vi "运维调试_五参数.vi"(11 "编号":string) -> ()   [LabVIEW 2016, in "斯坦道多参数.lvlib"]
uses:
  <vilib>/Utility/miscctls.llb/LVPointTypeDef.ctl
  <vilib>/Plasmionique/MB Master/MB_Master/MB_Master.lvclass
  <vilib>/Utility/config.llb/NI_LVConfig.lvlib
panel:
  in  "水样测量时间":dbl caption="水样测量时间:"
  in  "自动断线重连":bool=TRUE
  in  "打开modbus":bool
  out "选项卡控件":enum32{"选项卡 1", "选项卡 2"}(tab)
  in  "VISA资源名称":refnum<visa-resource-name> caption="串口"
  in  "IP":string="localhost" caption="IP:"
  in  "Port":u16=502 caption="Port:"
  in  "连接方式":u16(ring) items=["Modbus RTU", "Modbus TCP"]
  in  "藻密度校准":bool
  in  "权限2":bool
  out "权限1":bool
  out "密码":dbl
  in  "密码锁":bool
  in  "藻密度探头选择":u16(ring) items=["YL型", "MQ型", "NAQ型"]
  in  "叶绿素a探头选择":u16(ring) items=["YL型", "MQ型", "NAQ型"]
  in  "浊度探头选择":u16(ring) items=["YL型", "MQ型", "NAQ型"]
  in  "电导率探头选择":u16(ring) items=["YL型", "MQ型", "NAQ型"]
  in  "DO探头选择":u16(ring) items=["YL型", "MQ型", "NAQ型"]
  in  "pH探头选择":u16(ring) items=["YL型", "MQ型", "NAQ型"]
  in  "设置页返回":bool
  in  "藻密度":bool
  in  "叶绿素a启用":bool
  in  "Temp":bool
  in  "Cond":bool
  in  "Turb":bool
  in  "DO":bool
  in  "pH":bool
  in  "周期设置":bool
  out "当前串口":string
  out "运行状态":u16(ring) items=["空闲", "水样测试", "标样核查"]
  in  "叶绿素a校准":bool
  in  "停止":bool
  in  "标样核查":bool
  in  "水样测试":bool
  in  "设置":bool
  in  "水温校准":bool
  in  "浊度校准":bool
  in  "溶解氧校准":bool
  in  "电导率校准":bool
  in  "pH校准":bool
  in  "探头校正返回":bool
  in  "探头校正":bool
  out "检测值":T1(array[cluster])
  # "请设置仪器连接方式"
  # "请选择要启用的参数"
  # "min"
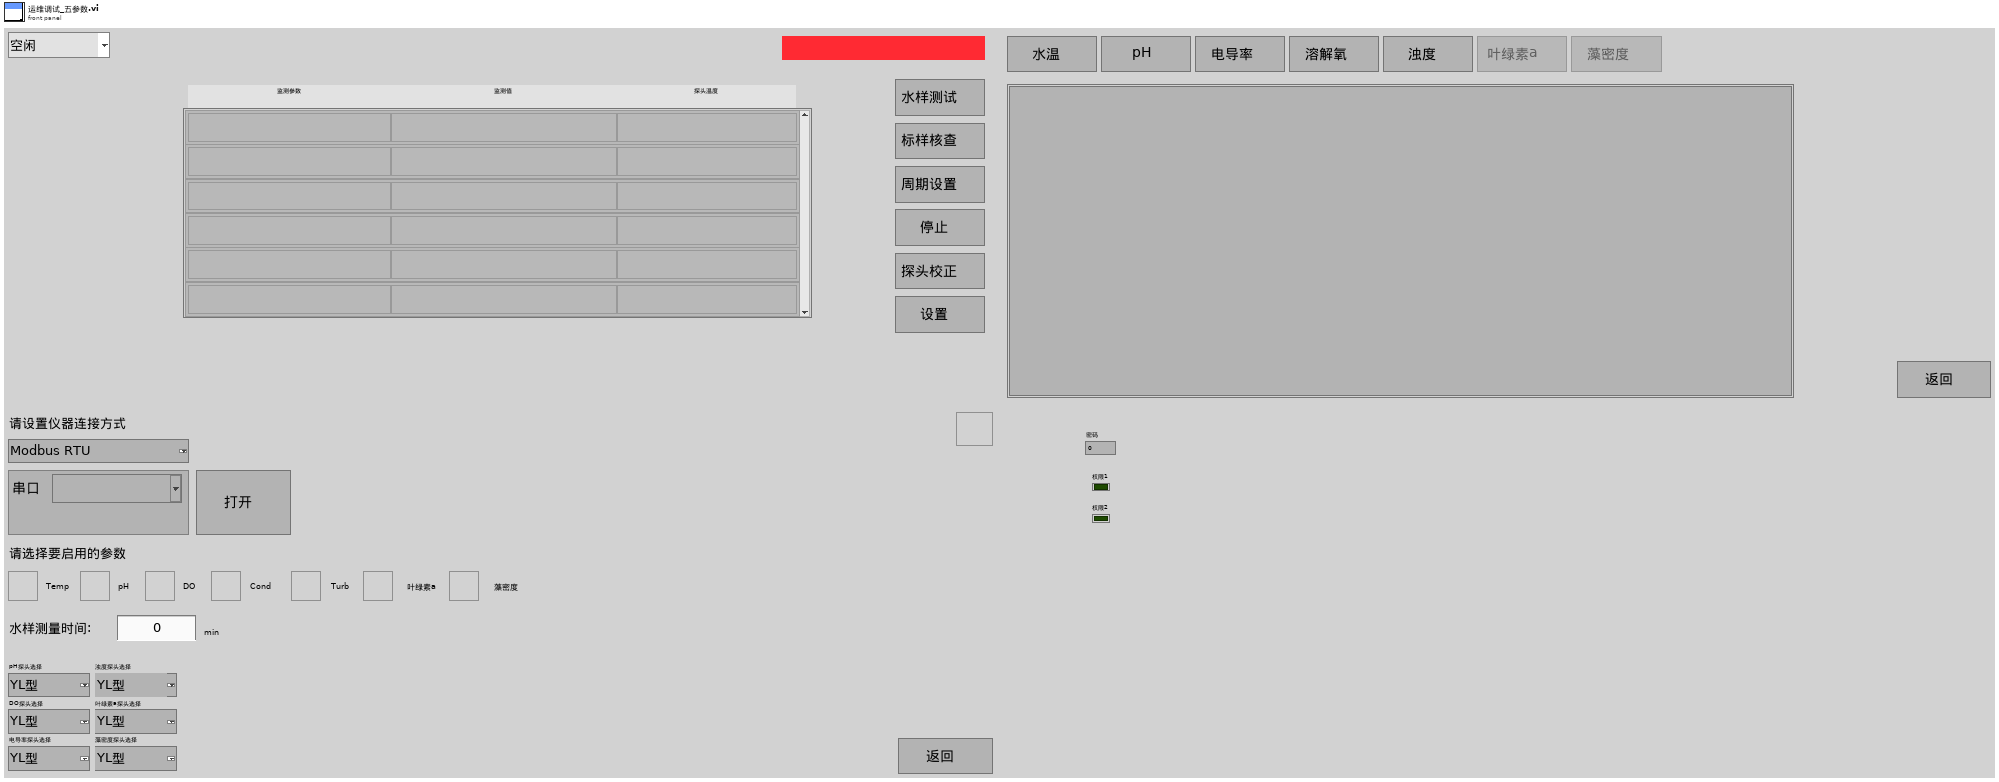
[diagram p1: front panel]
types:
  T1 = cluster{"监测参数1":string, "浓度1":string, "探头温度1":string}[]
  T2 = typedef "LVPointTypeDef.ctl" = cluster{"Horizontal":i16, "Vertical":i16}
  T3 = cluster{"温度测量值":sgl, "DO%":sgl, "DOmg/L":sgl, "温度偏移修正值":sgl}
  T4 = enum8{"Enabled", "Disabled", "Disabled and Grayed Out"}
  T5 = cluster{"pH探头选择":u16, "DO探头选择":u16, "电导率探头选择":u16, "浊度探头选择":u16, "叶绿素a探头选择":u16, "蓝绿藻探头选择":u16}
  T6 = cluster{"周期设置类型":enum16{"定点启动", "间隔启动"}, "定时功能启用":bool, "定时间隔":u32, "24H周期设置":bool[]}
  T7 = enum32{"Bad", "Idle", "Run top level", "Running"}
  T8 = typedef "LVDateTimeRec.ctl" = cluster{"秒数的小数部分":dbl, "秒":i32, "分":i32, "时":i32, "日":i32, "月":i32, "年":i32, "天数（周）":i32, "天数（年）":i32, "DST":i32}
  T9 = typedef "Semaphore RefNum" = refnum<k1>
  T10 = cluster{"电极状态标志":u16, "电极型号标志":u16, "溶解氧测量值":sgl, "温度测量值":sgl, "溶解氧饱和度值":sgl, "盐度补偿值":sgl, "大气压补偿值":sgl, "溶解氧偏移修正值":sgl, "温度偏移修正值":sgl, "手动温度补偿值":sgl, "溶解氧电极零点":sgl, "溶解氧电极斜率":sgl, "第1点标准值记录":sgl, "第1点信号值记录":sgl, "第1点温度值记录":sgl, "第2点标准值记录":sgl, "第2点信号值记录":sgl, "第2点温度值记录":sgl, "命令滤波设定":u16, "温度模式":enum16{"ATC", "MTC"}, "生产批次":u16, "电极序号":u16, "串口地址":u16, "串口波特率":enum16{"9600", "19200", "115200"}, "串口校验位":enum16{"NONE", "ODD", "EVEN"}, "串口停止位":enum16{"1bit", "2bit"}, "第一点标准值":sgl, "第二点标准值":sgl}
  T11 = cluster{"报警码":u16, "溶解氧数值（mg/L）":sgl, "溶解氧数据（%）":sgl, "温度数据":sgl, "溶解氧原始信号 nA":sgl, "大气压力":sgl, "盐度":sgl, "0X0009_NC":string, "产品名称":string, "序列号":string, "硬件版本":string, "软件版本":string, "通讯地址":u16, "波特率":u16, "设备类型":u16, "0X0026_NC":string, "第一点原始数据":sgl, "0X0033 NC":sgl, "第二点原始数据":sgl, "0X0037 NC":sgl, "探头校准命令":u16, "温度校准参数":sgl, "温度校准命令":u16}
  T12 = cluster{"电极状态标志":u16, "电极型号标志":u16, "酸碱度测量值":sgl, "温度测量值":sgl, "酸碱度信号值":sgl, "温度信号值":sgl, "酸碱度偏移修正值":sgl, "温度偏移修正值":sgl, "手动温度补偿值":sgl, "酸碱度电极零点":sgl, "酸碱度电极斜率":sgl, "第1点标准值记录":sgl, "第1点信号值记录":sgl, "第1点温度值记录":sgl, "第2点标准值记录":sgl, "第2点信号值记录":sgl, "第2点温度值记录":sgl, "命令滤波设定":u16, "温度模式":enum16{"ATC", "MTC"}, "生产批次":u16, "电极序号":u16, "串口地址":u16, "串口波特率":enum16{"9600", "19200", "115200"}, "串口校验位":enum16{"NONE", "ODD", "EVEN"}, "串口停止位":enum16{"1bit", "2bit"}, "第一点标准值":sgl, "第二点标准值":sgl}
  T13 = cluster{"报警码":u16, "pH数值":sgl, "0X0003_NC":sgl, "温度数据":sgl, "pH原始信号 mv":sgl, "0X0009_NC":string, "产品名称":string, "序列号":string, "硬件版本":string, "软件版本":string, "通讯地址":u16, "波特率":u16, "设备类型":u16, "0X0026_NC":string, "第一点原始数据":sgl, "第一点校准数据":sgl, "第二点原始数据":sgl, "第二点校准数据":sgl, "探头校准命令":u16, "温度校准参数":sgl, "温度校准命令":u16}
  T14 = cluster{"电极状态标志":u16, "电极型号标志":u16, "浊度测量值":sgl, "温度测量值":sgl, "浊度信号值":sgl, "浊度偏移修正值":sgl, "温度偏移修正值":sgl, "手动温度补偿值":sgl, "浊度电极零点":sgl, "浊度电极斜率":sgl, "第1点标准值记录":sgl, "第1点信号值记录":sgl, "第1点温度值记录":sgl, "第2点标准值记录":sgl, "第2点信号值记录":sgl, "第2点温度值记录":sgl, "命令滤波设定":u16, "温度模式":enum16{"ATC", "MTC"}, "生产批次":u16, "电极序号":u16, "串口地址":u16, "串口波特率":enum16{"9600", "19200", "115200"}, "串口校验位":enum16{"NONE", "ODD", "EVEN"}, "串口停止位":enum16{"1bit", "2bit"}, "第一点标准值":sgl, "第二点标准值":sgl, "第三点标准值":sgl}
  T15 = cluster{"报警码":u16, "浊度数值 NTU":sgl, "温度数据":sgl, "原始光强数值":u16, "量程":u16, "平均次数":u16, "清扫模式":u16, "清扫次数":u16, "清扫间隔分钟":u16, "0X000B_NC":string, "产品名称":string, "序列号":string, "硬件版本":string, "软件版本":string, "通讯地址":u16, "波特率":u16, "设备类型":u16, "0X0026_NC":string, "校准量程":u16, "第一点原始光强":u16, "第一点校准数据":sgl, "第二点原始光强":u16, "第二点校准数据":sgl, "第三点原始光强":u16, "第三点校准数据":sgl, "探头校准命令":u16, "温度校准参数":sgl, "温度校准命令":u16}
  T16 = cluster{"报警码":u16, "蓝绿藻":sgl, "温度数据":sgl, "原始光强数值":u16, "0X0006_NC":u16, "平均次数":u16, "清扫模式":u16, "清扫次数":u16, "清扫间隔分钟":u16, "0X000B_NC":string, "产品名称":string, "序列号":string, "硬件版本":string, "软件版本":string, "通讯地址":u16, "波特率":u16, "设备类型":u16, "0X0026_NC":string, "0X0030_NC":u16, "第一点原始光强":u16, "第一点校准数据":sgl, "第二点原始光强":u16, "第二点校准数据":sgl, "第三点原始光强":u16, "第三点校准数据":sgl, "探头校准命令":u16, "温度校准参数":sgl, "温度校准命令":u16}
  T17 = cluster{"报警码":u16, "叶绿素a":sgl, "温度数据":sgl, "原始光强数值":u16, "0X0006_NC":u16, "平均次数":u16, "清扫模式":u16, "清扫次数":u16, "清扫间隔分钟":u16, "0X000B_NC":string, "产品名称":string, "序列号":string, "硬件版本":string, "软件版本":string, "通讯地址":u16, "波特率":u16, "设备类型":u16, "0X0026_NC":string, "0X0030_NC":u16, "第一点原始光强":u16, "第一点校准数据":sgl, "第二点原始光强":u16, "第二点校准数据":sgl, "第三点原始光强":u16, "第三点校准数据":sgl, "探头校准命令":u16, "温度校准参数":sgl, "温度校准命令":u16}
  T18 = cluster{"电极状态标志":u16, "电极型号标志":u16, "电导率测量值":sgl, "温度测量值":sgl, "电导率信号值":sgl, "温度信号值":sgl, "温度补偿系数":sgl, "电导率偏移修正值":sgl, "温度偏移修正值":sgl, "手动温度补偿值":sgl, "电导率电极零点":sgl, "电导率电极斜率":sgl, "命令滤波设定":u16, "温度模式":enum16{"ATC", "MTC"}, "生产批次":u16, "电极序号":u16, "串口地址":u16, "串口波特率":enum16{"9600", "19200", "115200"}, "串口校验位":enum16{"NONE", "ODD", "EVEN"}, "串口停止位":enum16{"1bit", "2bit"}, "第一点标准值":sgl, "第二点标准值":sgl}
  T19 = cluster{"报警码":u16, "电导率数据（uS/cm）":sgl, "0x0003 NC":sgl, "温度数据":sgl, "电导率原始信号电阻":sgl, "当前量程":u16, "温度补偿系数":sgl, "0X0009_NC":string, "产品名称":string, "序列号":string, "硬件版本":string, "软件版本":string, "通讯地址":u16, "波特率":u16, "设备类型":u16, "0X0026_NC":string, "第一点原始数据":sgl, "第一点校准数据":sgl, "0X0035_NC":sgl, "0X0037_NC":sgl, "探头校准命令":u16, "温度校准参数":sgl, "温度校准命令":u16}
  T20 = typedef "NI_LVConfig.lvlib/Config Data RefNum.ctl" = refnum<k1>
  T21 = cluster{"pH校准VI引用句柄":refnum<vi>, "DO校准VI引用句柄":refnum<vi>, "COND校准VI引用句柄":refnum<vi>, "TURB校准VI引用句柄":refnum<vi>, "CHLA校准VI引用句柄":refnum<vi>, "BGA校准VI引用句柄":refnum<vi>}
  T22 = cluster{"数据保存间隔":dbl, "水温标样值":dbl, "pH标样值":dbl, "溶解氧标样值":dbl, "电导率标样值":dbl, "浊度标样值":dbl}
  T23 = cluster{"baud rate (bps)":u32, "stop bits":u16, "parity":u16, "flow control":u16, "timeout":u32, "retries":i32}
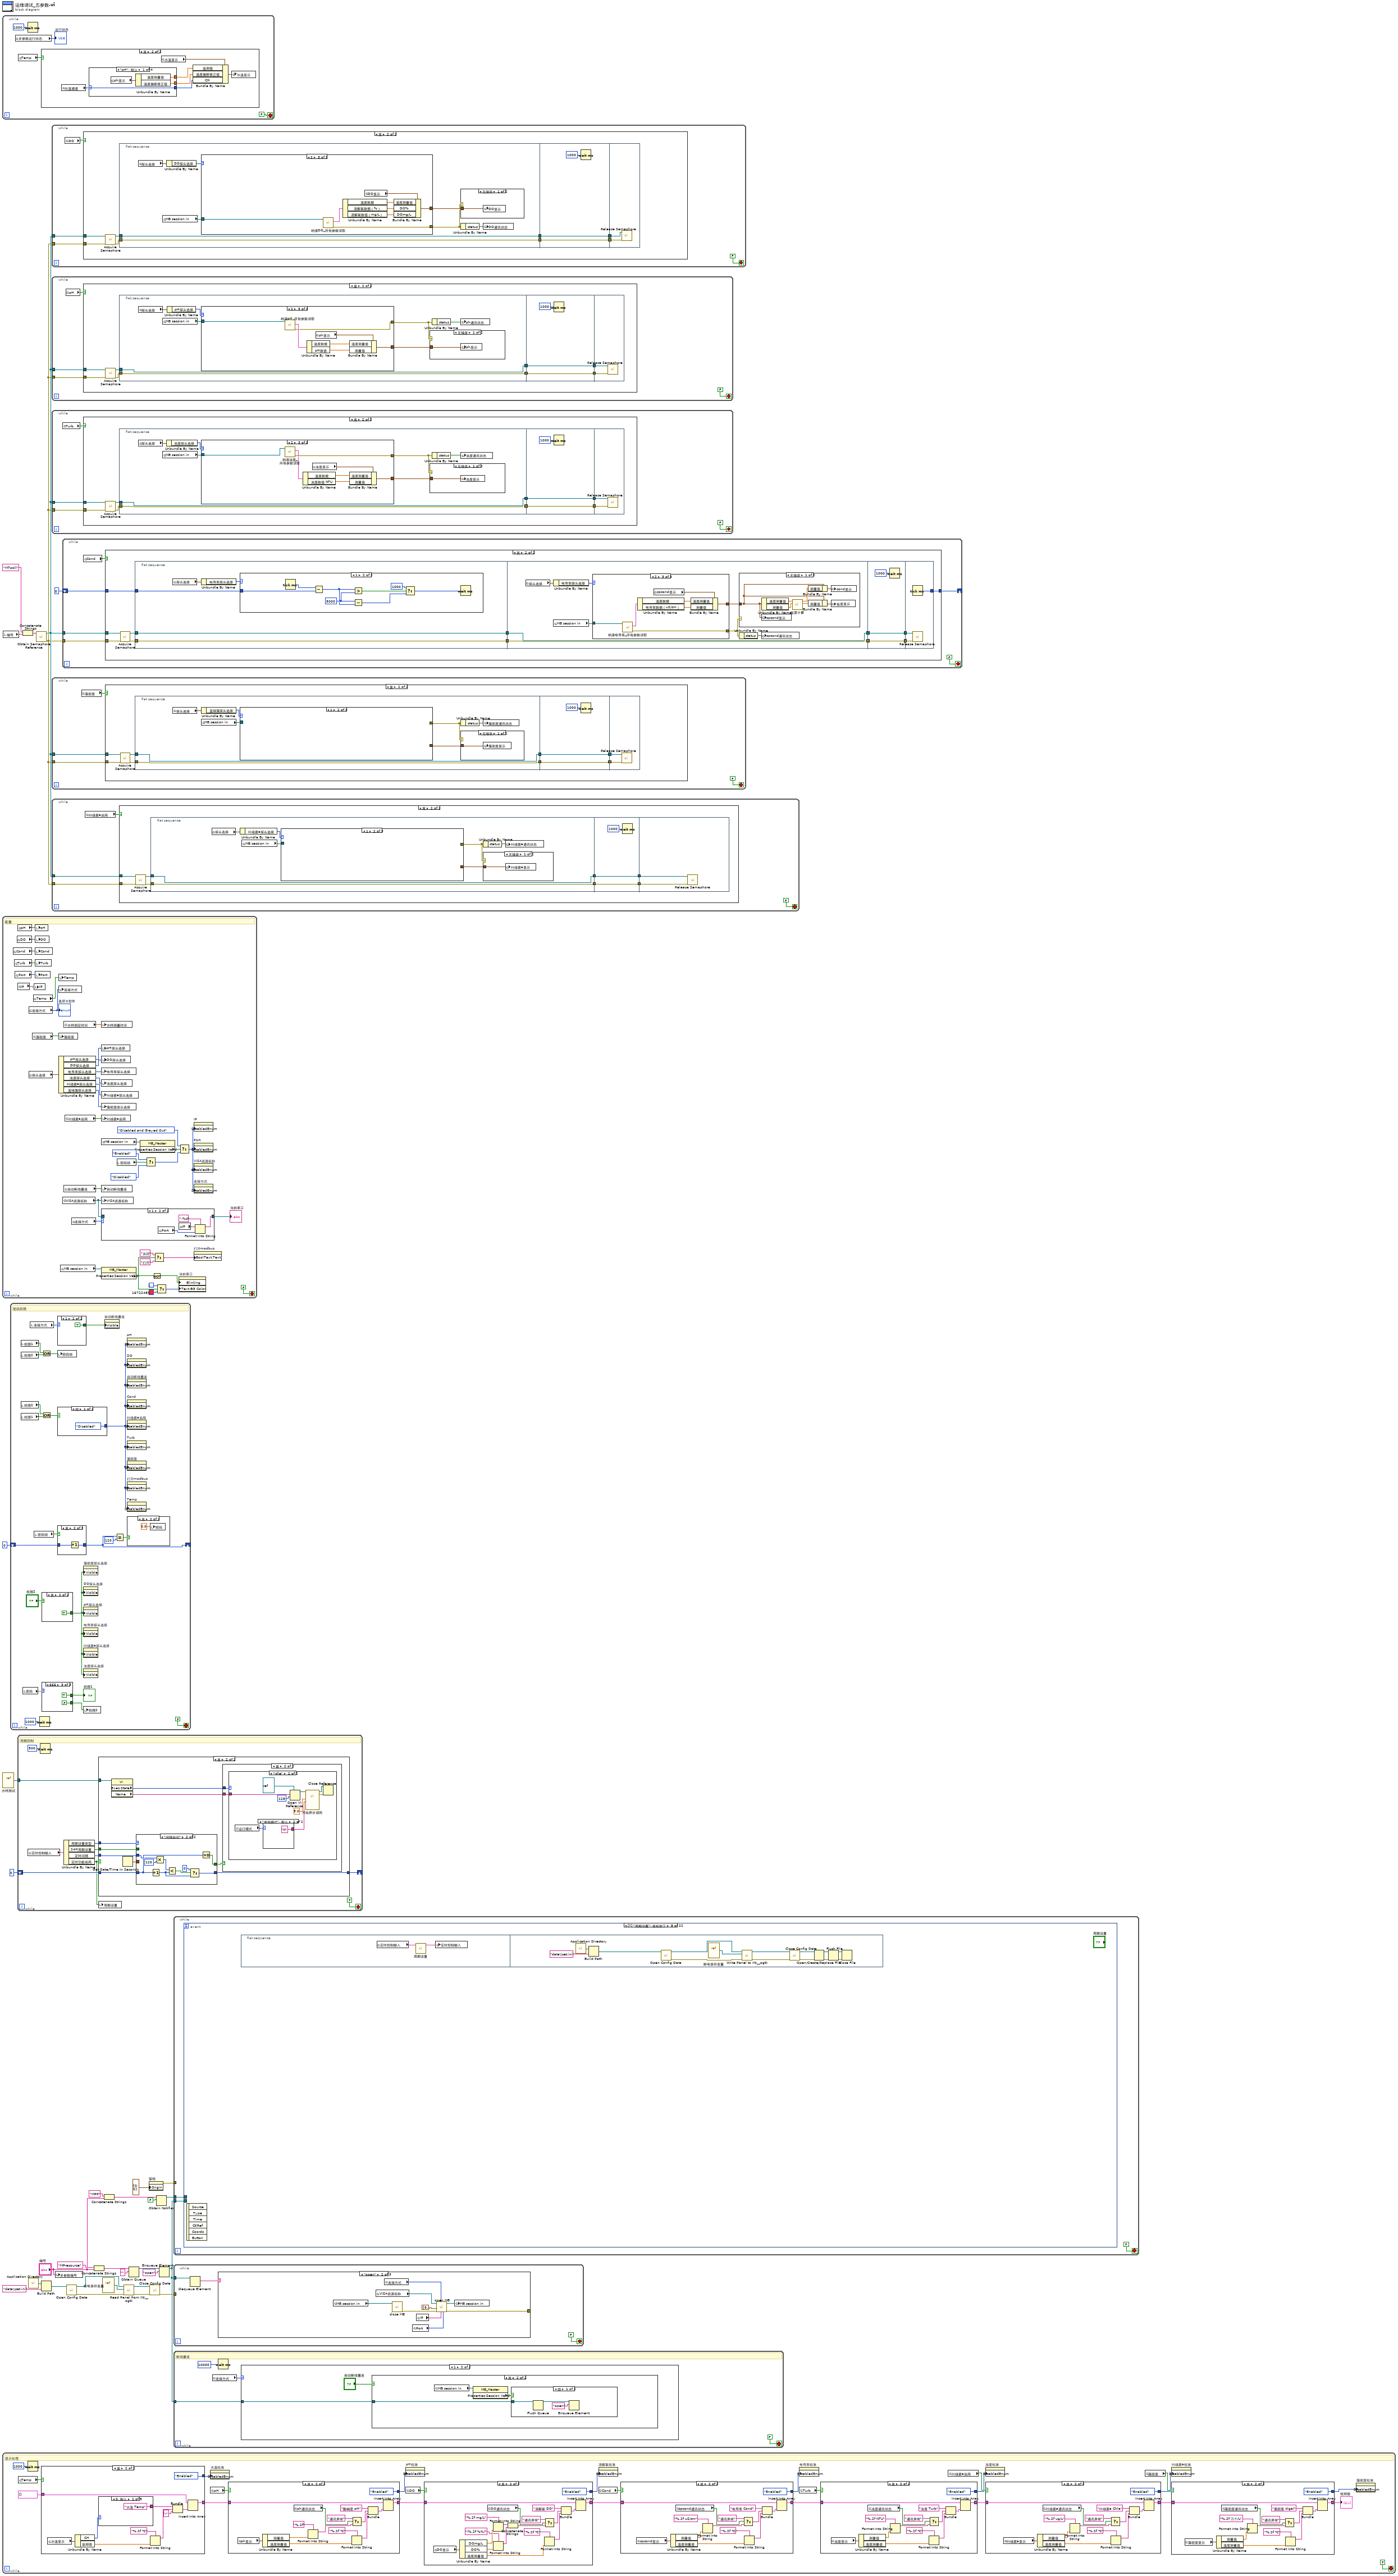
[diagram p0: block diagram]
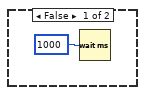
[diagram p5: hidden frame]
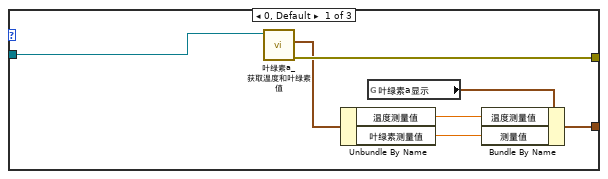
[diagram p6: hidden frame]
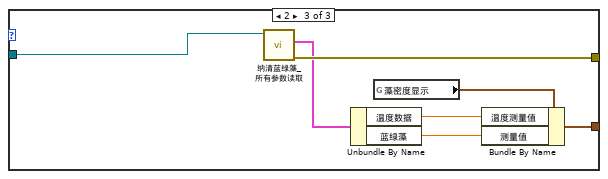
[diagram p7: hidden frame]
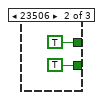
[diagram p13: hidden frame]
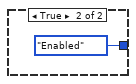
[diagram p14: hidden frame]
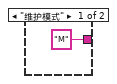
[diagram p19: hidden frame]
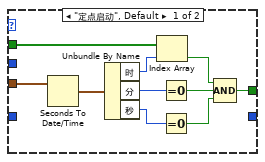
[diagram p20: hidden frame]
diagram:
  n1 = while {
    stop <- FALSE stop-if-true
    n2 = global read "多参数全局变量.vi" "多参数运行状态"() -> (→"运行状态":u16)
    n3 = global read "断电保存变量.vi" "Temp"() -> (w33:bool)
    n4 = Wait (ms)(milliseconds to wait=u32 1000 ("等待时间（毫秒）")) -> ()  [unwired: 1 out]
    n5 = case shown="真" w33 {
      frame False {
      }
      frame True {
        n6 = global read "断电保存变量.vi" "水温通道"() -> (w41:enum16{"pH", "Cond", "DO", "Turb"})
        n7 = case shown="\"pH\", 默认" w41 {
          selector: w41 -> [w45 w49 w53 w57]
          tunnel: [w45 w49 w53 w57] -> w40
          tunnel: [w43 w46 w50 w54] -> w39
          tunnel: [w44 w47 w51 w55] -> w38
          frame "pH", Default {
            n8 = global read "多参数全局变量.vi" "ph显示"() -> (w42:cluster{"温度测量值":sgl, "测量值":sgl, "温度偏移修正值":sgl})
            n9 = Unbundle By Name(w42) -> ("温度测量值"=w44:sgl, "温度偏移修正值"=w43:sgl)
          }
          frame "Cond" {
            n10 = global read "多参数全局变量.vi" "spcond显示"() -> (w48:cluster{"温度测量值":sgl, "测量值":sgl, "温度偏移修正值":sgl})
            n11 = Unbundle By Name(w48) -> ("温度测量值"=w47:sgl, "温度偏移修正值"=w46:sgl)
          }
          frame "DO" {
            n12 = global read "多参数全局变量.vi" "DO显示"() -> (w52:T3)
            n13 = Unbundle By Name(w52) -> ("温度测量值"=w51:sgl, "温度偏移修正值"=w50:sgl)
          }
          frame "Turb" {
            n14 = global read "多参数全局变量.vi" "浊度显示"() -> (w56:cluster{"温度测量值":sgl, "测量值":sgl, "温度偏移修正值":sgl})
            n15 = Unbundle By Name(w56) -> ("温度测量值"=w55:sgl, "温度偏移修正值"=w54:sgl)
          }
        }
        n16 = global read "多参数全局变量.vi" "水温显示"() -> (w36:cluster{"CH":u16, "监测值":dbl, "温度偏移修正值":sgl})
        n17 = Bundle By Name(cluster=w36, "监测值"=w38, "温度偏移修正值"=w39, "CH"=w40) -> (w37:cluster{"CH":u16, "监测值":dbl, "温度偏移修正值":sgl})
        n18 = global write "多参数全局变量.vi" "水温显示"(w37) -> ()
      }
    }
  }
  n19 = while {
    stop <- FALSE stop-if-true
    # "配置"
    n20 = global read "断电保存变量.vi" "Cond"() -> (w93:bool)
    n21 = global read "断电保存变量.vi" "Turb"() -> (w92:bool)
    n22 = global read "断电保存变量.vi" "Port"() -> (w71:u16)
    n23 = global read "断电保存变量.vi" "DO"() -> (w94:bool)
    n24 = global read "断电保存变量.vi" "pH"() -> (w95:bool)
    n25 = global read "断电保存变量.vi" "IP"() -> (w72:string)
    n26 = global read "断电保存变量.vi" "连接方式"() -> (w64:u16)
    "选项卡控件" <- w64
    n27 = global read "断电保存变量.vi" "探头选择"() -> (w82:T5)
    n28 = global read "断电保存变量.vi" "藻密度"() -> (w90:bool)
    n29 = global read "断电保存变量.vi" "Temp"() -> (w96:bool)
    n30 = local write "IP"(w72) -> ()
    n31 = local write "pH"(w95) -> ()
    n32 = local write "DO"(w94) -> ()
    n33 = local write "Cond"(w93) -> ()
    n34 = local write "Turb"(w92) -> ()
    n35 = local write "Port"(w71) -> ()
    n36 = local write "Temp"(w96) -> ()
    n37 = local write "连接方式"(w64) -> ()
    n38 = local write "藻密度"(w90) -> ()
    n39 = Unbundle By Name(w82) -> ("pH探头选择"=w65:u16, "DO探头选择"=w81:u16, "电导率探头选择"=w80:u16, "浊度探头选择"=w79:u16, "叶绿素a探头选择"=w78:u16, "蓝绿藻探头选择"=w77:u16)
    n40 = global read "多参数全局变量.vi" "MB session in"() -> (w86:refnum<class "MB_Master.lvclass">)
    n41 = global read "断电保存变量.vi" "VISA资源名称"() -> (w68:refnum<visa-resource-name>)
    n42 = global read "断电保存变量.vi" "水样测定时间"() -> (w58:dbl)
    n43 = global read "断电保存变量.vi" "自动断线重连"() -> (w59:bool)
    n44 = global read "断电保存变量.vi" "叶绿素a启用"() -> (w91:bool)
    n45 = global read "断电保存变量.vi" "连接方式"() -> (w69:u16)
    n46 = local write "水样测量时间"(w58) -> ()
    n47 = local write "pH探头选择"(w65) -> ()
    n48 = local write "DO探头选择"(w81) -> ()
    n49 = local write "电导率探头选择"(w80) -> ()
    n50 = local write "浊度探头选择"(w79) -> ()
    n51 = local write "叶绿素a探头选择"(w78) -> ()
    n52 = local write "藻密度探头选择"(w77) -> ()
    n53 = local write "叶绿素a启用"(w91) -> ()
    n54 = global read "多参数全局变量.vi" "MB session in"() -> (w89:refnum<class "MB_Master.lvclass">)
    n55 = local write "自动断线重连"(w59) -> ()
    n56 = local write "VISA资源名称"(w68) -> ()
    n57 = case shown="1" w69 {
      tunnel: w68 -> [w98 _]
      tunnel: [w98 w99] -> w67
      frame 0, Default {
      }
      frame 1 {
        n58 = global read "断电保存变量.vi" "Port"() -> (w100:u16)
        n59 = global read "断电保存变量.vi" "IP"() -> (w102:string)
        n60 = Format Into String(format string=":%d" ("格式字符串"), initial string=w102, w100) -> (resulting string=w99:string)  [unwired: 1 in, 1 out]
      }
    }
    "当前串口" <- w67
    n61 = property class="MB_Master"(reference=w86) -> ("Properties:Session Valid"=w63:bool)  [unwired: 1 in, 2 out]
    n62 = local read "密码锁"() -> (w76:bool)
    n63 = property class="MB_Master"(reference=w89) -> ("Properties:Session Valid"=w88:bool)  [unwired: 1 in, 2 out]
    n64 = Select(t=T4."Enabled" ("f"), s=w76, f=T4."Disabled") -> (s? t:f=w74:T4)
    n65 = Not(x=w63) -> (.not. x?=w66:bool)
    n66 = Select(t="关闭" ("布尔文本.文本"), s=w63, f="打开" ("布尔文本.文本")) -> (s? t:f=w83:string)
    n67 = Select(t=u32 16777216, s=w63, f=u32 16722483) -> (s? t:f=w60:u32)
    n68 = property on="当前串口" class="Str"("Blinking"=w66, "Text.BG Color"=w60) -> ()  [unwired: 2 in, 2 out]
    n69 = Select(t=T4."Disabled and Grayed Out" ("禁用"), s=w88, f=w74) -> (s? t:f=w70:T4)
    n70 = property on="IP" class="Str"("DisabledEnum"=w70) -> ()  [unwired: 2 in, 2 out]
    n71 = property on="Port" class="DigNum (严格)"("DisabledEnum"=w70) -> ()  [unwired: 2 in, 2 out]
    n72 = property on="VISA资源名称" class="VISAName"("DisabledEnum"=w70) -> ()  [unwired: 2 in, 2 out]
    n73 = property on="连接方式" class="Ring (严格)"("DisabledEnum"=w70) -> ()  [unwired: 2 in, 2 out]
    n74 = property on="打开modbus" class="Bool"("BoolText.Text"=w83) -> ()  [unwired: 2 in, 2 out]
  }
  n75 = vi-ref "水样测试.vi"() -> (w20:refnum<vi>)
  n76 = while {
    stop <- FALSE stop-if-true
    # "显示处理"
    n77 = global read "断电保存变量.vi" "Temp"() -> (w124:bool)
    n78 = Wait (ms)(milliseconds to wait=u32 1000 ("等待时间（毫秒）")) -> ()  [unwired: 1 out]
    n79 = case shown="真" w124 {
      tunnel: [w234 w239] -> w121
      tunnel: T1 [] ("数组") -> [w234 w240]
      tunnel: [T4."Disabled and Grayed Out" ("禁用") T4."Enabled" ("禁用")] -> w107
      frame False {
      }
      frame True {
        n80 = global read "多参数全局变量.vi" "水温显示"() -> (w237:cluster{"CH":u16, "监测值":dbl, "温度偏移修正值":sgl})
        n81 = Unbundle By Name(w237) -> ("CH"=w236:u16, "监测值"=w235:dbl)
        n82 = case shown="0, 默认" w236 {
          tunnel: ["水温 Temp" ("监测参数1") "水温 Temp (pH)" ("监测参数1") "水温 Temp (Cond)" ("监测参数1") "水温 Temp (DO)" ("监测参数1") "水温 Temp (Turb)" ("监测参数1")] -> w244
          frame 0, Default {
          }
          frame 1 {
          }
          frame 2 {
          }
          frame 3 {
          }
          frame 4 {
          }
        }
        n83 = Format Into String(format string="%.2f ℃" ("格式字符串"), w235) -> (resulting string=w243:string)  [unwired: 2 in, 1 out]
        n84 = Bundle("监测参数1"=w244, w243, "探头温度1"="-") -> (w241:cluster{"监测参数1":string, string, "探头温度1":string})  [unwired: 1 in]
        n85 = Insert Into Array(array=w240, new element=w241) -> (w239:T1)  [unwired: 1 in]
      }
    }
    n86 = property on="水温校准" class="Bool"("DisabledEnum"=w107) -> ()  [unwired: 2 in, 2 out]
    n87 = global read "断电保存变量.vi" "pH"() -> (w122:bool)
    n88 = case shown="真" w122 {
      tunnel: [w217 w224] -> w119
      tunnel: w121 -> [w217 w226]
      tunnel: [T4."Disabled and Grayed Out" ("禁用") T4."Enabled" ("禁用")] -> w112
      frame False {
      }
      frame True {
        n89 = global read "多参数全局变量.vi" "ph显示"() -> (w222:cluster{"温度测量值":sgl, "测量值":sgl, "温度偏移修正值":sgl})
        n90 = Unbundle By Name(w222) -> ("测量值"=w232:sgl, "温度测量值"=w230:sgl)
        n91 = global read "多参数全局变量.vi" "ph通讯状态"() -> (w220:bool)
        n92 = Format Into String(format string="%.2f" ("格式字符串"), w232) -> (resulting string=w219:string)  [unwired: 2 in, 1 out]
        n93 = Select(t="通讯异常" ("格式字符串"), s=w220, f=w219) -> (s? t:f=w218:string)
        n94 = Format Into String(format string="%.2f ℃" ("格式字符串"), w230) -> (resulting string=w228:string)  [unwired: 2 in, 1 out]
        n95 = Bundle("监测参数2"="酸碱度 pH", "格式字符串"=w218, w228) -> (w225:cluster{"监测参数2":string, "格式字符串":string, string})  [unwired: 1 in]
        n96 = Insert Into Array(array=w226, new element=w225) -> (w224:T1)  [unwired: 1 in]
      }
    }
    n97 = property on="pH校准" class="Bool"("DisabledEnum"=w112) -> ()  [unwired: 2 in, 2 out]
    n98 = global read "断电保存变量.vi" "DO"() -> (w120:bool)
    n99 = case shown="真" w120 {
      tunnel: [w196 w203] -> w116
      tunnel: w119 -> [w196 w204]
      tunnel: [T4."Disabled and Grayed Out" ("禁用") T4."Enabled" ("禁用")] -> w111
      frame False {
      }
      frame True {
        n100 = global read "多参数全局变量.vi" "DO显示"() -> (w201:T3)
        n101 = Unbundle By Name(w201) -> ("DOmg/L"=w212:sgl, "DO%"=w210:sgl, "温度测量值"=w214:sgl)
        n102 = global read "多参数全局变量.vi" "DO通讯状态"() -> (w199:bool)
        n103 = Format Into String(format string="%.2f mg/L" ("格式字符串"), w212) -> (resulting string=w209:string)  [unwired: 2 in, 1 out]
        n104 = Format Into String(format string="(%.2f %%)" ("格式字符串"), w210) -> (resulting string=w208:string)  [unwired: 2 in, 1 out]
        n105 = Concatenate Strings(w209, w208) -> (w198:string)
        n106 = Select(t="通讯异常" ("格式字符串"), s=w199, f=w198) -> (s? t:f=w197:string)
        n107 = Format Into String(format string="%.2f ℃" ("格式字符串"), w214) -> (resulting string=w206:string)  [unwired: 2 in, 1 out]
        n108 = Bundle("监测参数2"="溶解氧 DO", "格式字符串"=w197, w206) -> (w205:cluster{"监测参数2":string, "格式字符串":string, string})  [unwired: 1 in]
        n109 = Insert Into Array(array=w204, new element=w205) -> (w203:T1)  [unwired: 1 in]
      }
    }
    n110 = property on="溶解氧校准" class="Bool"("DisabledEnum"=w111) -> ()  [unwired: 2 in, 2 out]
    n111 = global read "断电保存变量.vi" "Cond"() -> (w118:bool)
    n112 = case shown="真" w118 {
      tunnel: w116 -> [w179 w190]
      tunnel: [w179 w188] -> w115
      tunnel: [T4."Disabled and Grayed Out" ("禁用") T4."Enabled" ("禁用")] -> w110
      frame False {
      }
      frame True {
        n113 = global read "多参数全局变量.vi" "spcond显示"() -> (w186:cluster{"温度测量值":sgl, "测量值":sgl, "温度偏移修正值":sgl})
        n114 = Unbundle By Name(w186) -> ("测量值"=w185:sgl, "温度测量值"=w184:sgl)
        n115 = global read "多参数全局变量.vi" "spcond通讯状态"() -> (w182:bool)
        n116 = Format Into String(format string="%.2f uS/cm" ("格式字符串"), w185) -> (resulting string=w181:string)  [unwired: 2 in, 1 out]
        n117 = Select(t="通讯异常" ("格式字符串"), s=w182, f=w181) -> (s? t:f=w180:string)
        n118 = Format Into String(format string="%.2f ℃" ("格式字符串"), w184) -> (resulting string=w191:string)  [unwired: 2 in, 1 out]
        n119 = Bundle("监测参数2"="电导率 Cond", "格式字符串"=w180, w191) -> (w189:cluster{"监测参数2":string, "格式字符串":string, string})  [unwired: 1 in]
        n120 = Insert Into Array(array=w190, new element=w189) -> (w188:T1)  [unwired: 1 in]
      }
    }
    n121 = property on="电导率校准" class="Bool"("DisabledEnum"=w110) -> ()  [unwired: 2 in, 2 out]
    n122 = global read "断电保存变量.vi" "Turb"() -> (w117:bool)
    n123 = case shown="真" w117 {
      tunnel: w115 -> [w162 w173]
      tunnel: [w162 w171] -> w114
      tunnel: [T4."Disabled and Grayed Out" ("禁用") T4."Enabled" ("禁用")] -> w109
      frame False {
      }
      frame True {
        n124 = global read "多参数全局变量.vi" "浊度显示"() -> (w169:cluster{"温度测量值":sgl, "测量值":sgl, "温度偏移修正值":sgl})
        n125 = Unbundle By Name(w169) -> ("测量值"=w168:sgl, "温度测量值"=w167:sgl)
        n126 = global read "多参数全局变量.vi" "浊度通讯状态"() -> (w165:bool)
        n127 = Format Into String(format string="%.2f NTU" ("格式字符串"), w168) -> (resulting string=w164:string)  [unwired: 2 in, 1 out]
        n128 = Select(t="通讯异常" ("格式字符串"), s=w165, f=w164) -> (s? t:f=w163:string)
        n129 = Format Into String(format string="%.2f ℃" ("格式字符串"), w167) -> (resulting string=w175:string)  [unwired: 2 in, 1 out]
        n130 = Bundle("监测参数2"="浊度 Turb", "格式字符串"=w163, w175) -> (w172:cluster{"监测参数2":string, "格式字符串":string, string})  [unwired: 1 in]
        n131 = Insert Into Array(array=w173, new element=w172) -> (w171:T1)  [unwired: 1 in]
      }
    }
    n132 = global read "断电保存变量.vi" "叶绿素a启用"() -> (w113:bool)
    n133 = property on="浊度校准" class="Bool"("DisabledEnum"=w109) -> ()  [unwired: 2 in, 2 out]
    n134 = case shown="真" w113 {
      tunnel: w114 -> [w145 w156]
      tunnel: [w145 w154] -> w104
      tunnel: [T4."Disabled and Grayed Out" ("禁用") T4."Enabled" ("禁用")] -> w108
      frame False {
      }
      frame True {
        n135 = global read "多参数全局变量.vi" "叶绿素a显示"() -> (w150:cluster{"温度测量值":sgl, "测量值":sgl, "温度偏移修正值":sgl})
        n136 = Unbundle By Name(w150) -> ("测量值"=w153:sgl, "温度测量值"=w152:sgl)
        n137 = global read "多参数全局变量.vi" "叶绿素a通讯状态"() -> (w148:bool)
        n138 = Format Into String(format string="%.2f ug/L" ("格式字符串"), w153) -> (resulting string=w147:string)  [unwired: 2 in, 1 out]
        n139 = Select(t="通讯异常" ("格式字符串"), s=w148, f=w147) -> (s? t:f=w146:string)
        n140 = Format Into String(format string="%.2f ℃" ("格式字符串"), w152) -> (resulting string=w158:string)  [unwired: 2 in, 1 out]
        n141 = Bundle("监测参数2"="叶绿素a Chla", "格式字符串"=w146, w158) -> (w155:cluster{"监测参数2":string, "格式字符串":string, string})  [unwired: 1 in]
        n142 = Insert Into Array(array=w156, new element=w155) -> (w154:T1)  [unwired: 1 in]
      }
    }
    n143 = global read "断电保存变量.vi" "藻密度"() -> (w105:bool)
    n144 = property on="叶绿素a校准" class="Bool"("DisabledEnum"=w108) -> ()  [unwired: 2 in, 2 out]
    n145 = case shown="真" w105 {
      tunnel: w104 -> [w128 w139]
      tunnel: [w128 w137] -> w103
      tunnel: [T4."Disabled and Grayed Out" ("禁用") T4."Enabled" ("禁用")] -> w106
      frame False {
      }
      frame True {
        n146 = global read "多参数全局变量.vi" "藻密度显示"() -> (w133:cluster{"温度测量值":sgl, "测量值":sgl, "温度偏移修正值":sgl})
        n147 = Unbundle By Name(w133) -> ("测量值"=w136:sgl, "温度测量值"=w135:sgl)
        n148 = global read "多参数全局变量.vi" "藻密度通讯状态"() -> (w131:bool)
        n149 = Format Into String(format string="%.2f 万个/L" ("格式字符串"), w136) -> (resulting string=w130:string)  [unwired: 2 in, 1 out]
        n150 = Select(t="通讯异常" ("格式字符串"), s=w131, f=w130) -> (s? t:f=w129:string)
        n151 = Format Into String(format string="%.2f ℃" ("格式字符串"), w135) -> (resulting string=w141:string)  [unwired: 2 in, 1 out]
        n152 = Bundle("监测参数2"="藻密度 Algal", "格式字符串"=w129, w141) -> (w138:cluster{"监测参数2":string, "格式字符串":string, string})  [unwired: 1 in]
        n153 = Insert Into Array(array=w139, new element=w138) -> (w137:T1)  [unwired: 1 in]
      }
    }
    "检测值" <- w103
    n154 = property on="藻密度校准" class="Bool"("DisabledEnum"=w106) -> ()  [unwired: 2 in, 2 out]
  }
  n155 = local read "编号"() -> (w16:string)
  n156 = while {
    shift-right: [w256] -> _
    shift-left: u32 0 ("等待时间（毫秒）") -> [w257]
    stop <- FALSE stop-if-true
    # "密码权限"
    n157 = local read "权限1"() -> (w262:bool)
    n158 = local read "权限2"() -> (w263:bool)
    n159 = local read "权限2"() -> (w260:bool)
    n160 = local read "权限1"() -> (w268:bool)
    n161 = local read "密码"() -> (w266:dbl)
    n162 = local read "连接方式"() -> (w253:u16)
    n163 = local read "密码锁"() -> (w258:bool)
    n164 = Wait (ms)(milliseconds to wait=u32 1000 ("等待时间（毫秒）")) -> ()  [unwired: 1 out]
    n165 = Or(x=w262, y=w263) -> (x .or. y?=w259:bool)
    n166 = Or(x=w260, y=w268) -> (x .or. y?=w261:bool)
    n167 = case shown="真" "权限2" {
      tunnel: [_ TRUE ("可见")] -> w270
      frame False {
      }
      frame True {
      }
    }
    n168 = case shown="666" w266 {
      tunnel: [_ TRUE ("可见") FALSE ("可见")] -> w265
      tunnel: [_ TRUE ("可见") TRUE ("可见")] -> w264
      frame 0, Default {
      }
      frame 23506 {
      }
      frame 666 {
      }
    }
    "权限1" <- w264
    n169 = case shown="1" w253 {
      tunnel: [_ TRUE ("可见")] -> w252
      frame 0, Default {
      }
      frame 1 {
      }
    }
    n170 = local write "密码锁"(w259) -> ()
    n171 = case shown="假" w261 {
      tunnel: [T4."Disabled" ("禁用") T4."Enabled" ("禁用")] -> w251
      frame False {
      }
      frame True {
      }
    }
    n172 = case shown="真" w258 {
      tunnel: w257 -> [_ w275]
      tunnel: [_ w274] -> w256
      frame False {
      }
      frame True {
        n173 = Increment(x=w275) -> (x+1=w274:u32)
      }
    }
    n174 = property on="藻密度探头选择" class="Ring (严格)"("Visible"=w270) -> ()  [unwired: 2 in, 2 out]
    n175 = property on="DO探头选择" class="Ring (严格)"("Visible"=w270) -> ()  [unwired: 2 in, 2 out]
    n176 = property on="pH探头选择" class="Ring (严格)"("Visible"=w270) -> ()  [unwired: 2 in, 2 out]
    n177 = property on="电导率探头选择" class="Ring (严格)"("Visible"=w270) -> ()  [unwired: 2 in, 2 out]
    n178 = property on="叶绿素a探头选择" class="Ring (严格)"("Visible"=w270) -> ()  [unwired: 2 in, 2 out]
    n179 = property on="浊度探头选择" class="Ring (严格)"("Visible"=w270) -> ()  [unwired: 2 in, 2 out]
    n180 = local write "权限2"(w265) -> ()
    n181 = property on="自动断线重连" class="Bool (严格)"("Visible"=w252) -> ()  [unwired: 2 in, 2 out]
    n182 = Greater Or Equal?(x=w256, y=u32 120) -> (x >= y?=w254:bool)
    n183 = property on="pH" class="Bool (严格)"("DisabledEnum"=w251) -> ()  [unwired: 2 in, 2 out]
    n184 = property on="DO" class="Bool (严格)"("DisabledEnum"=w251) -> ()  [unwired: 2 in, 2 out]
    n185 = property on="自动断线重连" class="Bool (严格)"("DisabledEnum"=w251) -> ()  [unwired: 2 in, 2 out]
    n186 = property on="Cond" class="Bool (严格)"("DisabledEnum"=w251) -> ()  [unwired: 2 in, 2 out]
    n187 = property on="叶绿素a启用" class="Bool (严格)"("DisabledEnum"=w251) -> ()  [unwired: 2 in, 2 out]
    n188 = property on="Turb" class="Bool (严格)"("DisabledEnum"=w251) -> ()  [unwired: 2 in, 2 out]
    n189 = property on="藻密度" class="Bool (严格)"("DisabledEnum"=w251) -> ()  [unwired: 2 in, 2 out]
    n190 = property on="打开modbus" class="Bool"("DisabledEnum"=w251) -> ()  [unwired: 2 in, 2 out]
    n191 = property on="Temp" class="Bool (严格)"("DisabledEnum"=w251) -> ()  [unwired: 2 in, 2 out]
    n192 = case shown="真" w254 {
      frame False {
      }
      frame True {
        n193 = local write "密码"(0.0 ("密码")) -> ()
      }
    }
  }
  n194 = while {
    tunnel: w20 -> [w285]
    shift-right: [w284] -> _
    shift-left: u32 0 ("等待时间（毫秒）") -> [w286]
    stop <- FALSE stop-if-true
    # "周期控制"
    n195 = global read "断电保存变量.vi" "定时控制输入"() -> (w288:T6)
    n196 = Wait (ms)(milliseconds to wait=u32 500 ("等待时间（毫秒）")) -> ()  [unwired: 1 out]
    n197 = Unbundle By Name(w288) -> ("周期设置类型"=w290:enum16{"定点启动", "间隔启动"}, "24H周期设置"=w289:bool[], "定时间隔"=w287:u32, "定时功能启用"=w283:bool)
    n198 = case shown="真" w283 {
      tunnel: w290 -> [_ w301]
      tunnel: w289 -> [_ w300]
      tunnel: w287 -> [_ w298]
      tunnel: w286 -> [_ w294]
      tunnel: w285 -> [_ w297]
      tunnel: [_ w293] -> w284
      frame False {
      }
      frame True {
        n199 = property class="VI"(reference=w297) -> ("Exec.State"=w295:T7, "Name"=w296:string)  [unwired: 1 in, 2 out]
        n200 = Get Date/Time In Seconds() -> (seconds since 1Jan1904=w302:timestamp)
        n201 = case shown="\"间隔启动\"" w301 {
          tunnel: w302 -> [w325 _]
          tunnel: w300 -> [w322 _]
          tunnel: [w316 w333] -> w299
          tunnel: w298 -> [_ w332]
          tunnel: w294 -> [_ w334]
          tunnel: [_ w328] -> w293
          frame "定点启动", Default {
            n202 = Seconds To Date/Time(time stamp (now)=w325) -> (date time rec=w324:T8)  [unwired: 1 in]
            n203 = Unbundle By Name(w324) -> ("时"=w323:i32, "分"=w321:i32, "秒"=w320:i32)
            n204 = Index Array(array=w322, index=w323) -> (element=w319:bool)
            n205 = Equal To 0?(x=w321) -> (x = 0?=w318:bool)
            n206 = Equal To 0?(x=w320) -> (x = 0?=w317:bool)
            n207 = Compound Arithmetic op=AND ("复合运算")(w319, w318, w317) -> (w316:bool)
          }
          frame "间隔启动" {
            n208 = Increment(x=w334) -> (x+1=w327:u32)
            n209 = Multiply(x=w332, y=u32 120) -> (x*y=w326:u32)
            n210 = Less?(x=w326, y=w327) -> (x < y?=w330:bool)
            n211 = Select(t=u32 0 ("y"), s=w330, f=w327) -> (s? t:f=w328:u32)
            n212 = Equal To 0?(x=w334) -> (x = 0?=w333:bool)
          }
        }
        n213 = case shown="真" w299 {
          tunnel: w295 -> [_ w304]
          tunnel: w296 -> [_ w303]
          frame False {
          }
          frame True {
            n214 = case shown="\"Idle\"" w304 {
              tunnel: w303 -> [_ w310]
              frame "Bad", Default {
              }
              frame "Idle" {
                n215 = global read "多参数全局变量.vi" "运行模式"() -> (w306:enum16{"维护模式", "常规模式", "应急模式", "质控模式"})
                n216 = case shown="\"常规模式\", 默认" w306 {
                  tunnel: ["M" ("数据标记表") "N" ("数据标记表")] -> w305
                  frame "维护模式" {
                  }
                  frame "常规模式", Default {
                  }
                }
                n217 = Open VI Reference(type specifier VI Refnum (for type only)=refnum<vi> refnum, vi path=w310, options=128 ("选项")) -> (vi reference=w311:refnum<vi>)  [unwired: 3 in, 1 out]
                n218 = call-by-ref "开始异步调用"(reference=w311, "数据标记表"=w305, "水样测试时间"=5.0) -> (reference out=w312:refnum<vi>, error out=w313:errorcluster)  [unwired: 11 in]
                n219 = Close Reference(reference=w312, error in (no error)=w313) -> ()  [unwired: 1 out]
              }
            }
          }
        }
      }
    }
    n220 = local write "周期设置"(w283) -> ()
  }
  n221 = Concatenate Strings("MTpoll" ("名称（未命名）"), w16) -> (w15:string)
  n222 = call <vilib>:"Application Directory.vi"() -> ("Application Directory"=w5:path)
  n223 = call <vilib>:"Obtain Semaphore Reference.vi"("name (unnamed)"=w15) -> ("error out"=w13:errorcluster, "semaphore"=w14:T9)  [unwired: 4 in, 1 out]
  n224 = Build Path(base path=w5, name or relative path="data\\set.ini" ("名称或相对路径")) -> (appended path=w4:path)
  n225 = while {
    tunnel: w14 -> [w336]
    tunnel: w13 -> [w335]
    stop <- FALSE stop-if-true
    n226 = global read "断电保存变量.vi" "DO"() -> (w337:bool)
    n227 = case shown="真" w337 {
      tunnel: w336 -> [_ w347]
      tunnel: w335 -> [_ w346]
      frame False {
        n228 = Wait (ms)(milliseconds to wait=u32 1000 ("等待时间（毫秒）")) -> ()  [unwired: 1 out]
      }
      frame True {
        n229 = call <vilib>:"Acquire Semaphore.vi"("error in (no error)"=w346, "semaphore"=w347) -> ("error out"=w344:errorcluster, "semaphore out"=w345:T9)  [unwired: 3 in, 1 out]
        n230 = flat-sequence {
          tunnel: w345 -> [w351]
          tunnel: [w351] -> w343
          tunnel: [w350] -> w341
          tunnel: w344 -> [w350]
          tunnel: w343 -> [w386]
          tunnel: [w386] -> w342
          tunnel: w341 -> [w385]
          tunnel: [w385] -> w340
          tunnel: w342 -> [w388]
          tunnel: w340 -> [w387]
          frame #0 {
            n231 = global read "断电保存变量.vi" "探头选择"() -> (w355:T5)
            n232 = global read "多参数全局变量.vi" "MB session in"() -> (w352:refnum<class "MB_Master.lvclass">)
            n233 = Unbundle By Name(w355) -> ("DO探头选择"=w354:u16)
            n234 = case shown="2" w354 {
              tunnel: w352 -> [w364 w374 w377]
              tunnel: [w362 w372 w381] -> w353
              tunnel: [w358 w367 w375] -> w349
              frame 0, Default {
                n235 = global read "断电保存变量.vi" "大气压补偿"() -> (w365:dbl)
                n236 = global read "断电保存变量.vi" "盐度补偿"() -> (w366:dbl)
                n237 = call "禹山溶解氧_获取温度和测量值.vi"("大气压补偿"=w365, "盐度补偿"=w366, "MB session in"=w364) -> ("error out"=w358:errorcluster, "输出值"=w356:cluster{"温度测量值":sgl, "DO%":sgl, "DOmg/L":sgl})  [unwired: 6 in, 1 out]
                n238 = global read "断电保存变量.vi" "DO温度偏移补偿"() -> (w357:dbl)
                n239 = Unbundle By Name(w356) -> ("温度测量值"=w361:sgl, "DO%"=w360:sgl, "DOmg/L"=w359:sgl)
                n240 = global read "多参数全局变量.vi" "DO显示"() -> (w363:T3)
                n241 = Bundle By Name(cluster=w363, "温度测量值"=w361, "DO%"=w360, "DOmg/L"=w359, "温度偏移修正值"=w357) -> (w362:T3)
              }
              frame 1 {
                n242 = call "DO_所有参数读取.vi"("MB session in"=w374) -> ("error out"=w367:errorcluster, "输出值"=w371:T10)  [unwired: 8 in, 1 out]
                n243 = Unbundle By Name(w371) -> ("温度测量值"=w368:sgl, "溶解氧饱和度值"=w369:sgl, "溶解氧测量值"=w370:sgl)
                n244 = global read "多参数全局变量.vi" "DO显示"() -> (w373:T3)
                n245 = Bundle By Name(cluster=w373, "温度测量值"=w368, "DO%"=w369, "DOmg/L"=w370) -> (w372:T3)
              }
              frame 2 {
                n246 = call "纳清DO_所有参数读取.vi"("MB session in"=w377) -> ("error out"=w375:errorcluster, "输出值"=w376:T11)  [unwired: 8 in, 1 out]
                n247 = Unbundle By Name(w376) -> ("温度数据"=w378:sgl, "溶解氧数据（%）"=w379:sgl, "溶解氧数值（mg/L）"=w380:sgl)
                n248 = global read "多参数全局变量.vi" "DO显示"() -> (w382:T3)
                n249 = Bundle By Name(cluster=w382, "温度测量值"=w378, "DO%"=w379, "DOmg/L"=w380) -> (w381:T3)
              }
            }
            n250 = case shown="无错误" w349 {
              tunnel: w353 -> [w383 _]
              frame No Error {
                n251 = global write "多参数全局变量.vi" "DO显示"(w383) -> ()
              }
              frame Error {
              }
            }
            n252 = Unbundle By Name(w349) -> ("status"=w348:bool)
            n253 = global write "多参数全局变量.vi" "DO通讯状态"(w348) -> ()
          }
          frame #1 {
            n254 = Wait (ms)(milliseconds to wait=u32 1000 ("等待时间（毫秒）")) -> ()  [unwired: 1 out]
          }
          frame #2 {
            n255 = call <vilib>:"Release Semaphore.vi"("error in (no error)"=w387, "semaphore"=w388) -> ()  [unwired: 4 in, 2 out]
          }
        }
      }
    }
  }
  n256 = while {
    tunnel: w14 -> [w390]
    tunnel: w13 -> [w389]
    stop <- FALSE stop-if-true
    n257 = global read "断电保存变量.vi" "pH"() -> (w391:bool)
    n258 = case shown="真" w391 {
      tunnel: w390 -> [_ w401]
      tunnel: w389 -> [_ w400]
      frame False {
        n259 = Wait (ms)(milliseconds to wait=u32 1000 ("等待时间（毫秒）")) -> ()  [unwired: 1 out]
      }
      frame True {
        n260 = call <vilib>:"Acquire Semaphore.vi"("error in (no error)"=w400, "semaphore"=w401) -> ("error out"=w394:errorcluster, "semaphore out"=w399:T9)  [unwired: 3 in, 1 out]
        n261 = flat-sequence {
          tunnel: w399 -> [w406]
          tunnel: [w406] -> w398
          tunnel: [w405] -> w395
          tunnel: w394 -> [w405]
          tunnel: w398 -> [w436]
          tunnel: [w436] -> w397
          tunnel: [w435] -> w396
          tunnel: w395 -> [w435]
          tunnel: w397 -> [w438]
          tunnel: w396 -> [w437]
          frame #0 {
            n262 = global read "断电保存变量.vi" "探头选择"() -> (w409:T5)
            n263 = global read "多参数全局变量.vi" "MB session in"() -> (w407:refnum<class "MB_Master.lvclass">)
            n264 = Unbundle By Name(w409) -> ("pH探头选择"=w408:u16)
            n265 = case shown="2" w408 {
              tunnel: w407 -> [w417 w425 w430]
              tunnel: [w416 w424 w428] -> w403
              tunnel: [w414 w421 w431] -> w404
              frame 0, Default {
                n266 = call "禹山pH_获取温度和测量值.vi"("MB session in"=w417) -> ("error out"=w416:errorcluster, "输出值"=w413:cluster{"温度测量值":sgl, "ORP":sgl, "pH":sgl})  [unwired: 8 in, 1 out]
                n267 = global read "断电保存变量.vi" "pH温度偏移补偿"() -> (w410:dbl)
                n268 = Unbundle By Name(w413) -> ("温度测量值"=w412:sgl, "pH"=w411:sgl)
                n269 = global read "多参数全局变量.vi" "ph显示"() -> (w415:cluster{"温度测量值":sgl, "测量值":sgl, "温度偏移修正值":sgl})
                n270 = Bundle By Name(cluster=w415, "温度测量值"=w412, "测量值"=w411, "温度偏移修正值"=w410) -> (w414:cluster{"温度测量值":sgl, "测量值":sgl, "温度偏移修正值":sgl})
              }
              frame 1 {
                n271 = call "pH_所有参数读取.vi"("MB session in"=w425) -> ("error out"=w424:errorcluster, "输出值"=w423:T12)  [unwired: 8 in, 1 out]
                n272 = Unbundle By Name(w423) -> ("温度测量值"=w418:sgl, "酸碱度测量值"=w419:sgl, "温度偏移修正值"=w420:sgl)
                n273 = global read "多参数全局变量.vi" "ph显示"() -> (w422:cluster{"温度测量值":sgl, "测量值":sgl, "温度偏移修正值":sgl})
                n274 = Bundle By Name(cluster=w422, "温度测量值"=w418, "测量值"=w419, "温度偏移修正值"=w420) -> (w421:cluster{"温度测量值":sgl, "测量值":sgl, "温度偏移修正值":sgl})
              }
              frame 2 {
                n275 = call "纳清pH_所有参数读取.vi"("MB session in"=w430) -> ("error out"=w428:errorcluster, "输出值"=w429:T13)  [unwired: 8 in, 1 out]
                n276 = Unbundle By Name(w429) -> ("温度数据"=w427:sgl, "pH数值"=w426:sgl)
                n277 = global read "多参数全局变量.vi" "ph显示"() -> (w432:cluster{"温度测量值":sgl, "测量值":sgl, "温度偏移修正值":sgl})
                n278 = Bundle By Name(cluster=w432, "温度测量值"=w427, "测量值"=w426) -> (w431:cluster{"温度测量值":sgl, "测量值":sgl, "温度偏移修正值":sgl})
              }
            }
            n279 = case shown="无错误" w403 {
              tunnel: w404 -> [w433 _]
              frame No Error {
                n280 = global write "多参数全局变量.vi" "ph显示"(w433) -> ()
              }
              frame Error {
              }
            }
            n281 = Unbundle By Name(w403) -> ("status"=w402:bool)
            n282 = global write "多参数全局变量.vi" "ph通讯状态"(w402) -> ()
          }
          frame #1 {
            n283 = Wait (ms)(milliseconds to wait=u32 1000 ("等待时间（毫秒）")) -> ()  [unwired: 1 out]
          }
          frame #2 {
            n284 = call <vilib>:"Release Semaphore.vi"("error in (no error)"=w437, "semaphore"=w438) -> ()  [unwired: 4 in, 2 out]
          }
        }
      }
    }
  }
  n285 = while {
    tunnel: w14 -> [w440]
    tunnel: w13 -> [w439]
    stop <- FALSE stop-if-true
    n286 = global read "断电保存变量.vi" "Turb"() -> (w441:bool)
    n287 = case shown="真" w441 {
      tunnel: w440 -> [_ w451]
      tunnel: w439 -> [_ w450]
      frame False {
        n288 = Wait (ms)(milliseconds to wait=u32 1000 ("等待时间（毫秒）")) -> ()  [unwired: 1 out]
      }
      frame True {
        n289 = call <vilib>:"Acquire Semaphore.vi"("error in (no error)"=w450, "semaphore"=w451) -> ("error out"=w444:errorcluster, "semaphore out"=w447:T9)  [unwired: 3 in, 1 out]
        n290 = flat-sequence {
          tunnel: [w455] -> w448
          tunnel: w447 -> [w455]
          tunnel: [w454] -> w445
          tunnel: w444 -> [w454]
          tunnel: [w485] -> w449
          tunnel: w448 -> [w485]
          tunnel: [w484] -> w446
          tunnel: w445 -> [w484]
          tunnel: w449 -> [w487]
          tunnel: w446 -> [w486]
          frame #0 {
            n291 = global read "断电保存变量.vi" "探头选择"() -> (w459:T5)
            n292 = global read "多参数全局变量.vi" "MB session in"() -> (w456:refnum<class "MB_Master.lvclass">)
            n293 = Unbundle By Name(w459) -> ("浊度探头选择"=w458:u16)
            n294 = case shown="2" w458 {
              tunnel: w456 -> [w467 w474 w477]
              tunnel: [w465 w469 w478] -> w457
              tunnel: [w464 w468 w476] -> w453
              frame 0, Default {
                n295 = call "禹山浊度_获取温度和测量值.vi"("MB session in"=w467) -> ("error out"=w464:errorcluster, "输出值"=w463:cluster{"温度测量值":sgl, "浊度":sgl})  [unwired: 8 in, 1 out]
                n296 = global read "断电保存变量.vi" "Turb温度偏移补偿"() -> (w460:dbl)
                n297 = Unbundle By Name(w463) -> ("温度测量值"=w462:sgl, "浊度"=w461:sgl)
                n298 = global read "多参数全局变量.vi" "浊度显示"() -> (w466:cluster{"温度测量值":sgl, "测量值":sgl, "温度偏移修正值":sgl})
                n299 = Bundle By Name(cluster=w466, "温度测量值"=w462, "测量值"=w461, "温度偏移修正值"=w460) -> (w465:cluster{"温度测量值":sgl, "测量值":sgl, "温度偏移修正值":sgl})
              }
              frame 1 {
                n300 = call "浊度_所有参数读取.vi"("MB session in"=w474) -> ("error out"=w468:errorcluster, "输出值"=w473:T14)  [unwired: 8 in, 1 out]
                n301 = Unbundle By Name(w473) -> ("温度测量值"=w471:sgl, "浊度测量值"=w470:sgl)
                n302 = global read "多参数全局变量.vi" "浊度显示"() -> (w472:cluster{"温度测量值":sgl, "测量值":sgl, "温度偏移修正值":sgl})
                n303 = Bundle By Name(cluster=w472, "温度测量值"=w471, "测量值"=w470) -> (w469:cluster{"温度测量值":sgl, "测量值":sgl, "温度偏移修正值":sgl})
              }
              frame 2 {
                n304 = call "纳清浊度_所有参数读取.vi"("MB session in"=w477) -> ("error out"=w476:errorcluster, "输出值"=w475:T15)  [unwired: 8 in, 1 out]
                n305 = Unbundle By Name(w475) -> ("温度数据"=w480:sgl, "浊度数值 NTU"=w479:sgl)
                n306 = global read "多参数全局变量.vi" "浊度显示"() -> (w481:cluster{"温度测量值":sgl, "测量值":sgl, "温度偏移修正值":sgl})
                n307 = Bundle By Name(cluster=w481, "温度测量值"=w480, "测量值"=w479) -> (w478:cluster{"温度测量值":sgl, "测量值":sgl, "温度偏移修正值":sgl})
              }
            }
            n308 = case shown="无错误" w453 {
              tunnel: w457 -> [w482 _]
              frame No Error {
                n309 = global write "多参数全局变量.vi" "浊度显示"(w482) -> ()
              }
              frame Error {
              }
            }
            n310 = Unbundle By Name(w453) -> ("status"=w452:bool)
            n311 = global write "多参数全局变量.vi" "浊度通讯状态"(w452) -> ()
          }
          frame #1 {
            n312 = Wait (ms)(milliseconds to wait=u32 1000 ("等待时间（毫秒）")) -> ()  [unwired: 1 out]
          }
          frame #2 {
            n313 = call <vilib>:"Release Semaphore.vi"("error in (no error)"=w486, "semaphore"=w487) -> ()  [unwired: 4 in, 2 out]
          }
        }
      }
    }
  }
  n314 = while {
    tunnel: w14 -> [w489]
    tunnel: w13 -> [w488]
    stop <- FALSE stop-if-true
    n315 = global read "断电保存变量.vi" "藻密度"() -> (w490:bool)
    n316 = case shown="真" w490 {
      tunnel: w489 -> [_ w500]
      tunnel: w488 -> [_ w499]
      frame False {
        n317 = Wait (ms)(milliseconds to wait=u32 1000 ("等待时间（毫秒）")) -> ()  [unwired: 1 out]
      }
      frame True {
        n318 = call <vilib>:"Acquire Semaphore.vi"("error in (no error)"=w499, "semaphore"=w500) -> ("error out"=w494:errorcluster, "semaphore out"=w496:T9)  [unwired: 3 in, 1 out]
        n319 = flat-sequence {
          tunnel: [w504] -> w497
          tunnel: w496 -> [w504]
          tunnel: [w503] -> w495
          tunnel: w494 -> [w503]
          tunnel: [w525] -> w498
          tunnel: w497 -> [w525]
          tunnel: w495 -> [w524]
          tunnel: [w524] -> w493
          tunnel: w498 -> [w528]
          tunnel: w493 -> [w527]
          frame #0 {
            n320 = global read "断电保存变量.vi" "探头选择"() -> (w507:T5)
            n321 = Unbundle By Name(w507) -> ("蓝绿藻探头选择"=w506:u16)
            n322 = global read "多参数全局变量.vi" "MB session in"() -> (w505:refnum<class "MB_Master.lvclass">)
            n323 = case shown="1" w506 {
              tunnel: [w515 _ w520] -> w502
              tunnel: w505 -> [w514 _ w522]
              tunnel: [w512 _ w519] -> w508
              frame 0, Default {
                n324 = call "叶绿素a_获取温度和叶绿素值.vi"("MB session in"=w514) -> ("error out"=w515:errorcluster, "输出值"=w511:cluster{"温度测量值":sgl, "叶绿素测量值":sgl, "错误标志":u16})  [unwired: 8 in, 1 out]
                n325 = Unbundle By Name(w511) -> ("温度测量值"=w509:sgl, "叶绿素测量值"=w510:sgl)
                n326 = global read "多参数全局变量.vi" "叶绿素a显示"() -> (w513:cluster{"温度测量值":sgl, "测量值":sgl, "温度偏移修正值":sgl})
                n327 = Bundle By Name(cluster=w513, "温度测量值"=w509, "测量值"=w510) -> (w512:cluster{"温度测量值":sgl, "测量值":sgl, "温度偏移修正值":sgl})
              }
              frame 1 {
              }
              frame 2 {
                n328 = call "纳清蓝绿藻_所有参数读取.vi"("MB session in"=w522) -> ("error out"=w520:errorcluster, "输出值"=w518:T16)  [unwired: 8 in, 1 out]
                n329 = Unbundle By Name(w518) -> ("温度数据"=w516:sgl, "蓝绿藻"=w517:sgl)
                n330 = global read "多参数全局变量.vi" "藻密度显示"() -> (w521:cluster{"温度测量值":sgl, "测量值":sgl, "温度偏移修正值":sgl})
                n331 = Bundle By Name(cluster=w521, "温度测量值"=w516, "测量值"=w517) -> (w519:cluster{"温度测量值":sgl, "测量值":sgl, "温度偏移修正值":sgl})
              }
            }
            n332 = Unbundle By Name(w502) -> ("status"=w501:bool)
            n333 = case shown="无错误" w502 {
              tunnel: w508 -> [w523 _]
              frame No Error {
                n334 = global write "多参数全局变量.vi" "藻密度显示"(w523) -> ()
              }
              frame Error {
              }
            }
            n335 = global write "多参数全局变量.vi" "藻密度通讯状态"(w501) -> ()
          }
          frame #1 {
            n336 = Wait (ms)(milliseconds to wait=u32 1000 ("等待时间（毫秒）")) -> ()  [unwired: 1 out]
          }
          frame #2 {
            n337 = call <vilib>:"Release Semaphore.vi"("error in (no error)"=w527, "semaphore"=w528) -> ()  [unwired: 4 in, 2 out]
          }
        }
      }
    }
  }
  n338 = while {
    tunnel: w14 -> [w530]
    tunnel: w13 -> [w529]
    stop <- FALSE stop-if-true
    n339 = global read "断电保存变量.vi" "叶绿素a启用"() -> (w531:bool)
    n340 = case shown="真" w531 {
      tunnel: w530 -> [_ w539]
      tunnel: w529 -> [_ w535]
      frame False {
        n341 = Wait (ms)(milliseconds to wait=u32 1000 ("等待时间（毫秒）")) -> ()  [unwired: 1 out]
      }
      frame True {
        n342 = call <vilib>:"Acquire Semaphore.vi"("error in (no error)"=w535, "semaphore"=w539) -> ("error out"=w534:errorcluster, "semaphore out"=w536:T9)  [unwired: 3 in, 1 out]
        n343 = flat-sequence {
          tunnel: [w545] -> w540
          tunnel: w536 -> [w545]
          tunnel: [w544] -> w537
          tunnel: w534 -> [w544]
          tunnel: [w567] -> w541
          tunnel: w540 -> [w567]
          tunnel: [w566] -> w538
          tunnel: w537 -> [w566]
          tunnel: w541 -> [w569]
          tunnel: w538 -> [w568]
          frame #0 {
            n344 = global read "断电保存变量.vi" "探头选择"() -> (w548:T5)
            n345 = Unbundle By Name(w548) -> ("叶绿素a探头选择"=w547:u16)
            n346 = global read "多参数全局变量.vi" "MB session in"() -> (w546:refnum<class "MB_Master.lvclass">)
            n347 = case shown="1" w547 {
              tunnel: [w556 _ w561] -> w543
              tunnel: w546 -> [w555 _ w563]
              tunnel: [w553 _ w560] -> w549
              frame 0, Default {
                n348 = call "叶绿素a_获取温度和叶绿素值.vi"("MB session in"=w555) -> ("error out"=w556:errorcluster, "输出值"=w552:cluster{"温度测量值":sgl, "叶绿素测量值":sgl, "错误标志":u16})  [unwired: 8 in, 1 out]
                n349 = Unbundle By Name(w552) -> ("温度测量值"=w550:sgl, "叶绿素测量值"=w551:sgl)
                n350 = global read "多参数全局变量.vi" "叶绿素a显示"() -> (w554:cluster{"温度测量值":sgl, "测量值":sgl, "温度偏移修正值":sgl})
                n351 = Bundle By Name(cluster=w554, "温度测量值"=w550, "测量值"=w551) -> (w553:cluster{"温度测量值":sgl, "测量值":sgl, "温度偏移修正值":sgl})
              }
              frame 1 {
              }
              frame 2 {
                n352 = call "纳清叶绿素a_所有参数读取.vi"("MB session in"=w563) -> ("error out"=w561:errorcluster, "输出值"=w559:T17)  [unwired: 8 in, 1 out]
                n353 = global read "多参数全局变量.vi" "叶绿素a显示"() -> (w562:cluster{"温度测量值":sgl, "测量值":sgl, "温度偏移修正值":sgl})
                n354 = Unbundle By Name(w559) -> ("温度数据"=w557:sgl, "叶绿素a"=w558:sgl)
                n355 = Bundle By Name(cluster=w562, "温度测量值"=w557, "测量值"=w558) -> (w560:cluster{"温度测量值":sgl, "测量值":sgl, "温度偏移修正值":sgl})
              }
            }
            n356 = Unbundle By Name(w543) -> ("status"=w542:bool)
            n357 = case shown="无错误" w543 {
              tunnel: w549 -> [w564 _]
              frame No Error {
                n358 = global write "多参数全局变量.vi" "叶绿素a显示"(w564) -> ()
              }
              frame Error {
              }
            }
            n359 = global write "多参数全局变量.vi" "叶绿素a通讯状态"(w542) -> ()
          }
          frame #1 {
            n360 = Wait (ms)(milliseconds to wait=u32 1000 ("等待时间（毫秒）")) -> ()  [unwired: 1 out]
          }
          frame #2 {
            n361 = call <vilib>:"Release Semaphore.vi"("error in (no error)"=w568, "semaphore"=w569) -> ()  [unwired: 4 in, 2 out]
          }
        }
      }
    }
  }
  n362 = global write "多参数全局变量.vi" "多参数编号"("编号") -> ()
  n363 = while {
    tunnel: w14 -> [w573]
    tunnel: w13 -> [w572]
    shift-right: [w570] -> _
    shift-left: u32 0 ("millisecond timer value") -> [w571]
    stop <- FALSE stop-if-true
    n364 = global read "断电保存变量.vi" "Cond"() -> (w574:bool)
    n365 = case shown="真" w574 {
      tunnel: w573 -> [_ w588]
      tunnel: w572 -> [_ w587]
      tunnel: w571 -> [_ w578]
      tunnel: [_ w577] -> w570
      frame False {
        n366 = Wait (ms)(milliseconds to wait=u32 1000 ("等待时间（毫秒）")) -> ()  [unwired: 1 out]
      }
      frame True {
        n367 = call <vilib>:"Acquire Semaphore.vi"("error in (no error)"=w587, "semaphore"=w588) -> ("error out"=w582:errorcluster, "semaphore out"=w585:T9)  [unwired: 3 in, 1 out]
        n368 = flat-sequence {
          tunnel: w582 -> [w592]
          tunnel: w585 -> [w593]
          tunnel: [w593] -> w580
          tunnel: [w592] -> w579
          tunnel: w578 -> [w591]
          tunnel: [w605] -> w586
          tunnel: [w604] -> w583
          tunnel: w580 -> [w605]
          tunnel: w579 -> [w604]
          tunnel: w586 -> [w642]
          tunnel: [w642] -> w584
          tunnel: w583 -> [w641]
          tunnel: [w641] -> w581
          tunnel: w584 -> [w645]
          tunnel: w581 -> [w644]
          tunnel: [w643] -> w577
          frame #0 {
            n369 = global read "断电保存变量.vi" "探头选择"() -> (w590:T5)
            n370 = Unbundle By Name(w590) -> ("电导率探头选择"=w589:u16)
            n371 = case shown="1" w589 {
              tunnel: w591 -> [_ w596]
              frame 0, Default {
              }
              frame 1 {
                w599 = u32 5000 ("y")
                n372 = Tick Count (ms)() -> (millisecond timer value=w594:u32)
                n373 = Subtract(x=w594, y=w596) -> (x-y=w595:u32)
                n374 = Greater?(x=w595, y=w599) -> (0:w601:bool)
                n375 = Subtract(x=w599, y=w595) -> (x-y=w598:u32)
                n376 = Select(t=u32 1000 ("y"), s=w601, f=w598) -> (s? t:f=w597:u32)
                n377 = Wait (ms)(milliseconds to wait=w597) -> ()  [unwired: 1 out]
              }
            }
          }
          frame #1 {
            n378 = global read "断电保存变量.vi" "探头选择"() -> (w609:T5)
            n379 = Unbundle By Name(w609) -> ("电导率探头选择"=w608:u16)
            n380 = global read "多参数全局变量.vi" "MB session in"() -> (w606:refnum<class "MB_Master.lvclass">)
            n381 = case shown="2" w608 {
              tunnel: w606 -> [w617 w625 w628]
              tunnel: [w611 w623 w631] -> w607
              tunnel: [w616 w622 w626] -> w603
              frame 0, Default {
                n382 = call "禹山电导率_获取温度和测量值.vi"("MB session in"=w617) -> ("error out"=w616:errorcluster, "输出值"=w614:cluster{"温度测量值":sgl, "电导率":sgl, "错误标志":u16})  [unwired: 8 in, 1 out]
                n383 = global read "断电保存变量.vi" "Cond温度偏移补偿"() -> (w610:dbl)
                n384 = Unbundle By Name(w614) -> ("温度测量值"=w613:sgl, "电导率"=w612:sgl)
                n385 = global read "多参数全局变量.vi" "spcond显示"() -> (w615:cluster{"温度测量值":sgl, "测量值":sgl, "温度偏移修正值":sgl})
                n386 = Bundle By Name(cluster=w615, "温度测量值"=w613, "测量值"=w612, "温度偏移修正值"=w610) -> (w611:cluster{"温度测量值":sgl, "测量值":sgl, "温度偏移修正值":sgl})
              }
              frame 1 {
                n387 = call "电导率_所有参数读取.vi"("MB session in"=w625) -> ("error out"=w622:errorcluster, "输出值"=w621:T18)  [unwired: 8 in, 1 out]
                n388 = Unbundle By Name(w621) -> ("温度测量值"=w620:sgl, "电导率测量值"=w619:sgl, "电导率偏移修正值"=w618:sgl)
                n389 = global read "多参数全局变量.vi" "spcond显示"() -> (w624:cluster{"温度测量值":sgl, "测量值":sgl, "温度偏移修正值":sgl})
                n390 = Bundle By Name(cluster=w624, "温度测量值"=w620, "测量值"=w619, "温度偏移修正值"=w618) -> (w623:cluster{"温度测量值":sgl, "测量值":sgl, "温度偏移修正值":sgl})
              }
              frame 2 {
                n391 = call "纳清电导率_所有参数读取.vi"("MB session in"=w628) -> ("error out"=w626:errorcluster, "输出值"=w627:T19)  [unwired: 8 in, 1 out]
                n392 = Unbundle By Name(w627) -> ("温度数据"=w630:sgl, "电导率数据（uS/cm）"=w629:sgl)
                n393 = global read "多参数全局变量.vi" "spcond显示"() -> (w632:cluster{"温度测量值":sgl, "测量值":sgl, "温度偏移修正值":sgl})
                n394 = Bundle By Name(cluster=w632, "温度测量值"=w630, "测量值"=w629) -> (w631:cluster{"温度测量值":sgl, "测量值":sgl, "温度偏移修正值":sgl})
              }
            }
            n395 = case shown="无错误" w603 {
              tunnel: w607 -> [w634 _]
              frame No Error {
                n396 = Unbundle By Name(w634) -> ("温度测量值"=w639:sgl, "测量值"=w638:sgl)
                n397 = global write "多参数全局变量.vi" "spcond显示"(w634) -> ()
                n398 = call "盐度计算.vi"("spCond"=w638, "Temp"=w639) -> ("saltresult"=w633:dbl, "cond"=w637:dbl)  [unwired: 8 in]
                n399 = Bundle By Name(cluster=w634, "测量值"=w637) -> (w636:cluster{"温度测量值":sgl, "测量值":sgl, "温度偏移修正值":sgl})
                n400 = Bundle By Name(cluster=w634, "测量值"=w633) -> (w635:cluster{"温度测量值":sgl, "测量值":sgl, "温度偏移修正值":sgl})
                n401 = global write "多参数全局变量.vi" "cond显示"(w636) -> ()
                n402 = global write "多参数全局变量.vi" "盐度显示"(w635) -> ()
              }
              frame Error {
              }
            }
            n403 = Unbundle By Name(w603) -> ("status"=w602:bool)
            n404 = global write "多参数全局变量.vi" "spcond通讯状态"(w602) -> ()
          }
          frame #2 {
            n405 = Wait (ms)(milliseconds to wait=u32 1000 ("等待时间（毫秒）")) -> ()  [unwired: 1 out]
          }
          frame #3 {
            n406 = Tick Count (ms)() -> (millisecond timer value=w643:u32)
            n407 = call <vilib>:"Release Semaphore.vi"("error in (no error)"=w644, "semaphore"=w645) -> ()  [unwired: 4 in, 2 out]
          }
        }
      }
    }
  }
  n408 = call <vilib>:"Open Config Data.vi"("configuration file path"=w4) -> ("error out"=w8:errorcluster, "refnum"=w9:T20)  [unwired: 8 in, 1 out]
  n409 = Concatenate Strings("MPresource" ("名称（未命名）"), "编号") -> (w23:string)
  n410 = vi-ref "断电保存变量.vi"() -> (w2:refnum<vi>)
  n411 = Concatenate Strings("MPP" ("名称（未命名）"), "编号") -> (w24:string)
  n412 = call <userlib>:"Read Panel from INI__ogtk.vi"("error in (no error)"=w8, "VI ref"=w2, "refnum"=w9) -> ("error out"=w6:errorcluster, "refnum out"=w7:T20)  [unwired: 7 in]
  n413 = Obtain Queue(name (unnamed)=w23, element data type="" ("名称（未命名）")) -> (queue out=w18:refnum<queue>)  [unwired: 3 in, 2 out]
  n414 = property on="窗格" class="Pane"("Origin"=T2 {"Horizontal"=0, "Vertical"=0} ("原点")) -> (error out=w31:errorcluster)  [unwired: 2 in, 1 out]
  n415 = call <vilib>:"Close Config Data.vi"("error in (no error)"=w6, "refnum"=w7) -> ("error out"=w1:errorcluster)  [unwired: 8 in, 1 out]
  n416 = Obtain Notifier(name (unnamed)=w24, notification data type=FALSE) -> (notifier out=w27:refnum<notifier>)  [unwired: 2 in, 2 out]
  n417 = Enqueue Element(queue=w18, element="open" ("元素")) -> (queue out=w11:refnum<queue>)  [unwired: 2 in, 2 out]
  n418 = while {
    tunnel: w31 -> [_]
    tunnel: w27 -> [w647]
    tunnel: w11 -> [w646]
    stop <- FALSE stop-if-true
    n419 = event shown="[7] \"周期设置\": 鼠标按下" {
      selector: _ -> [_ _ _ _ _ _ _ _ _ _ _ _ _ _ _ _ _ _ _ _ _ _]
      dyn-events: _ -> [_ _ _ _ _ _ _ _ _ _ _ _ _ _ _ _ _ _ _ _ _ _]
      timeout: _ -> [_ _ _ _ _ _ _ _ _ _ _ _ _ _ _ _ _ _ _ _ _ _]
      tunnel: w647 -> [_ _ _ _ _ _ _ _ _ _ w766 _ _ _ _ _ _ _ _ _ _ _]
      tunnel: w646 -> [_ _ _ _ _ _ _ _ _ _ _ _ _ w796 _ _ _ _ _ _ _ _]
      event Timeout {
        n420 = event-data() -> ()  [unwired: 1 in, 3 out]
      }
      event "水样测量时间": Mouse Down {
        n421 = event-data() -> ("CtlRef"=w649:refnum<vi>)  [unwired: 1 in, 5 out]
        n422 = property class="DigNum (严格)"(reference=w649) -> (reference out=w652:refnum<vi>, "Value"=w651:dbl)  [unwired: 1 in, 1 out]
        n423 = call "数字键盘.vi"("OldNumber"=w651) -> ("NewNumber"=w650:dbl)  [unwired: 1 in]
        n424 = property class="DigNum (严格)"(reference=w652, "Val(Sgnl)"=w650) -> ()  [unwired: 1 in, 2 out]
      }
      event "pH探头选择", "DO探头选择", "电导率探头选择", "浊度探头选择", "叶绿素a探头选择", "藻密度探头选择": Value Change {
        n425 = event-data() -> ("CtlRef"=w653:refnum<vi>, "NewVal"=w654:u16)  [unwired: 1 in, 4 out]
        n426 = Two Button Dialog(message="请再次确认修改的型号是否与实际匹配，否则将导致通讯异常，并且此操作将终止所有正在校准的参数！" ("消息")) -> (T button?=w655:bool)  [unwired: 2 in]
        n427 = case shown="真" w655 {
          tunnel: w654 -> [_ w658]
          tunnel: w653 -> [_ w657]
          frame False {
          }
          frame True {
            n428 = flat-sequence {
              tunnel: w658 -> [w659]
              tunnel: w657 -> [w663]
              frame #0 {
                n429 = property class="Ring (严格)"(reference=w663) -> ("Label.Text"=w662:string)  [unwired: 1 in, 2 out]
                n430 = global read "断电保存变量.vi" "探头选择"() -> (w661:T5)
                n431 = global read "多参数全局变量.vi" "校准VI引用句柄"() -> (w664:T21)
                n432 = case shown="\"蓝绿藻探头选择\"" w662 {
                  tunnel: w661 -> [w666 w669 w672 w675 w678 w681 w684]
                  tunnel: [w666 w668 w671 w674 w677 w680 w683] -> w660
                  tunnel: w659 -> [_ w667 w670 w673 w676 w679 w682]
                  frame Default {
                  }
                  frame "pH探头选择" {
                    n433 = Bundle By Name(cluster=w669, "pH探头选择"=w667) -> (w668:T5)
                  }
                  frame "电导率探头选择" {
                    n434 = Bundle By Name(cluster=w672, "电导率探头选择"=w670) -> (w671:T5)
                  }
                  frame "DO探头选择" {
                    n435 = Bundle By Name(cluster=w675, "DO探头选择"=w673) -> (w674:T5)
                  }
                  frame "浊度探头选择" {
                    n436 = Bundle By Name(cluster=w678, "浊度探头选择"=w676) -> (w677:T5)
                  }
                  frame "叶绿素a探头选择" {
                    n437 = Bundle By Name(cluster=w681, "叶绿素a探头选择"=w679) -> (w680:T5)
                  }
                  frame "蓝绿藻探头选择" {
                    n438 = Bundle By Name(cluster=w684, "蓝绿藻探头选择"=w682) -> (w683:T5)
                  }
                }
                n439 = Cluster To Array(cluster=w664) -> (array=w665:refnum<vi>[])
                n440 = for {
                  tunnel: w665 -> [w686] mode=indexing
                  tunnel: [w685] -> _ mode=indexing
                  n441 = invoke class="VI" method="Abort VI"(reference=w686) -> (error out=w685:errorcluster)  [unwired: 2 in, 2 out]
                }
                n442 = global write "断电保存变量.vi" "探头选择"(w660) -> ()
              }
              frame #1 {
                n443 = call <vilib>:"Application Directory.vi"() -> ("Application Directory"=w691:path)
                n444 = Build Path(base path=w691, name or relative path="data\\set.ini" ("名称或相对路径")) -> (appended path=w692:path)
                n445 = call <vilib>:"Open Config Data.vi"("configuration file path"=w692) -> ("error out"=w688:errorcluster, "refnum"=w687:T20)  [unwired: 8 in, 1 out]
                n446 = vi-ref "断电保存变量.vi"() -> (w694:refnum<vi>)
                n447 = call <userlib>:"Write Panel to INI__ogtk.vi"("error in (no error)"=w688, "VI ref"=w694, "refnum"=w687) -> ("error out"=w690:errorcluster, "refnum out"=w689:T20)  [unwired: 7 in]
                n448 = call <vilib>:"Close Config Data.vi"("error in (no error)"=w690, "refnum"=w689) -> ("error out"=w698:errorcluster, "file path"=w697:path)  [unwired: 8 in]
                n449 = Open/Create/Replace File(file path (use dialog)=w697, error in=w698) -> (refnum out=w696:refnum<file>, error out=w695:errorcluster)  [unwired: 4 in, 1 out]
                n450 = Flush File(refnum=w696, error in=w695) -> (refnum out=w700:refnum<file>, error out=w699:errorcluster)
                n451 = Close File(refnum=w700, error in=w699) -> ()  [unwired: 2 out]
              }
            }
          }
        }
      }
      event "VISA资源名称", "pH", "DO", "Turb", "Cond", "Temp", "叶绿素a启用", "打开modbus", "藻密度", "连接方式", "自动断线重连": Mouse Down {
        n452 = event-data() -> ()  [unwired: 1 in, 6 out]
        n453 = local read "密码锁"() -> (w701:bool)
        n454 = case shown="假" w701 {
          frame False {
            n455 = One Button Dialog(message="当前操作权限不足,请提升权限!!!" ("消息")) -> ()  [unwired: 1 in, 1 out]
          }
          frame True {
          }
        }
      }
      event "IP": Mouse Down {
        n456 = event-data() -> ("CtlRef"=w704:refnum<vi>)  [unwired: 1 in, 7 out]
        n457 = property on="IP" class="Str"() -> ("DisabledEnum"=w703:T4)  [unwired: 2 in, 2 out]
        n458 = case shown="\"Disabled and Grayed Out\"" w703 {
          tunnel: w704 -> [w708 _ _]
          frame "Enabled" {
            n459 = property class="Str"(reference=w708) -> (reference out=w707:refnum<vi>, "Value"=w706:string)  [unwired: 1 in, 1 out]
            n460 = call "字符键盘.vi"("Old String"=w706) -> ("String"=w705:string)  [unwired: 10 in]
            n461 = property class="Str"(reference=w707, "Val(Sgnl)"=w705) -> ()  [unwired: 1 in, 2 out]
          }
          frame "Disabled and Grayed Out" {
            n462 = One Button Dialog(message="关闭连接后才可设置!" ("消息")) -> ()  [unwired: 1 in, 1 out]
          }
          frame "Disabled", Default {
            n463 = One Button Dialog(message="当前操作权限不足,请提升权限!!!" ("消息")) -> ()  [unwired: 1 in, 1 out]
          }
        }
      }
      event "Port": Mouse Down {
        n464 = event-data() -> ("CtlRef"=w712:refnum<vi>)  [unwired: 1 in, 7 out]
        n465 = property on="Port" class="DigNum (严格)"() -> ("DisabledEnum"=w711:T4)  [unwired: 2 in, 2 out]
        n466 = case shown="\"Enabled\"" w711 {
          tunnel: w712 -> [w716 _ _]
          frame "Enabled" {
            n467 = property class="DigNum (严格)"(reference=w716) -> (reference out=w715:refnum<vi>, "Value"=w714:u16)  [unwired: 1 in, 1 out]
            n468 = call "数字键盘.vi"("OldNumber"=w714) -> ("NewNumber"=w713:dbl)  [unwired: 1 in]
            n469 = property class="DigNum (严格)"(reference=w715, "Val(Sgnl)"=w713) -> ()  [unwired: 1 in, 2 out]
          }
          frame "Disabled and Grayed Out" {
            n470 = One Button Dialog(message="关闭连接后才可设置!" ("消息")) -> ()  [unwired: 1 in, 1 out]
          }
          frame "Disabled", Default {
            n471 = One Button Dialog(message="当前操作权限不足,请提升权限!!!" ("消息")) -> ()  [unwired: 1 in, 1 out]
          }
        }
      }
      event "密码锁": Value Change {
        n472 = event-data() -> ("NewVal"=w719:bool)  [unwired: 1 in, 5 out]
        n473 = case shown="假" w719 {
          frame False {
            n474 = local write "密码"(0.0 ("密码")) -> ()
          }
          frame True {
            n475 = call "数字键盘.vi"("显示样式"=u32 2) -> ("NewNumber"=→"密码":dbl)  [unwired: 1 in]
          }
        }
      }
      event "周期设置": Mouse Down {
        n476 = event-data() -> ()  [unwired: 1 in, 6 out]
        n477 = flat-sequence {
          frame #0 {
            n478 = global read "断电保存变量.vi" "定时控制输入"() -> (w724:T6)
            n479 = call "周期设置.vi"("定时控制输入"=w724) -> ("定时控制输出"=w723:T6)  [unwired: 10 in]
            n480 = global write "断电保存变量.vi" "定时控制输入"(w723) -> ()
          }
          frame #1 {
            n481 = call <vilib>:"Application Directory.vi"() -> ("Application Directory"=w734:path)
            n482 = Build Path(base path=w734, name or relative path="data\\set.ini" ("名称或相对路径")) -> (appended path=w733:path)
            n483 = call <vilib>:"Open Config Data.vi"("configuration file path"=w733) -> ("error out"=w737:errorcluster, "refnum"=w738:T20)  [unwired: 8 in, 1 out]
            n484 = vi-ref "断电保存变量.vi"() -> (w731:refnum<vi>)
            n485 = call <userlib>:"Write Panel to INI__ogtk.vi"("error in (no error)"=w737, "VI ref"=w731, "refnum"=w738) -> ("error out"=w735:errorcluster, "refnum out"=w736:T20)  [unwired: 7 in]
            n486 = call <vilib>:"Close Config Data.vi"("error in (no error)"=w735, "refnum"=w736) -> ("error out"=w727:errorcluster, "file path"=w728:path)  [unwired: 8 in]
            n487 = Open/Create/Replace File(file path (use dialog)=w728, error in=w727) -> (refnum out=w729:refnum<file>, error out=w730:errorcluster)  [unwired: 4 in, 1 out]
            n488 = Flush File(refnum=w729, error in=w730) -> (refnum out=w725:refnum<file>, error out=w726:errorcluster)
            n489 = Close File(refnum=w725, error in=w726) -> ()  [unwired: 2 out]
          }
        }
      }
      event "水样测试": Value Change {
        n490 = event-data() -> ()  [unwired: 1 in, 6 out]
        n491 = vi-ref "水样测试.vi"() -> (w741:refnum<vi>)
        n492 = property class="VI"(reference=w741) -> ("Name"=w745:string, "Exec.State"=w743:T7)  [unwired: 1 in, 2 out]
        n493 = Open VI Reference(type specifier VI Refnum (for type only)=refnum<vi> refnum, vi path=w745, options=128 ("选项")) -> (vi reference=w746:refnum<vi>)  [unwired: 3 in, 1 out]
        n494 = case shown="\"Idle\"" w743 {
          tunnel: [w747 w750] -> w742
          tunnel: w746 -> [w747 w749]
          tunnel: "hd" ("数据标记表") -> [_ w748]
          frame "Bad", Default {
          }
          frame "Idle" {
            n495 = call-by-ref "开始异步调用"(reference=w749, "数据标记表"=w748) -> (reference out=w750:refnum<vi>)  [unwired: 12 in, 1 out]
          }
        }
        n496 = Close Reference(reference=w742) -> ()  [unwired: 1 in, 1 out]
      }
      event "标样核查": Value Change {
        n497 = event-data() -> ()  [unwired: 1 in, 6 out]
        n498 = call "标样核查配置.vi"() -> ("确认输出"=w752:bool, "标样核查配置"=w751:T22)  [unwired: 10 in]
        n499 = case shown="真" w752 {
          tunnel: w751 -> [_ w753]
          frame False {
          }
          frame True {
            n500 = vi-ref "标样核查.vi"() -> (w754:refnum<vi>)
            n501 = property class="VI"(reference=w754) -> ("Name"=w759:string, "Exec.State"=w756:T7)  [unwired: 1 in, 2 out]
            n502 = Open VI Reference(type specifier VI Refnum (for type only)=refnum<vi> refnum, vi path=w759, options=128 ("选项")) -> (vi reference=w760:refnum<vi>)  [unwired: 3 in, 1 out]
            n503 = case shown="\"Idle\"" w756 {
              tunnel: [w761 w764] -> w755
              tunnel: w760 -> [w761 w763]
              tunnel: w753 -> [_ w762]
              frame "Bad", Default {
              }
              frame "Idle" {
                n504 = call-by-ref "开始异步调用"(reference=w763, "标样核查配置"=w762) -> (reference out=w764:refnum<vi>)  [unwired: 12 in, 1 out]
              }
            }
            n505 = Close Reference(reference=w755) -> ()  [unwired: 1 in, 1 out]
          }
        }
      }
      event "停止": Value Change {
        n506 = event-data() -> ()  [unwired: 1 in, 6 out]
        n507 = Send Notification(notification=TRUE ("通知"), notifier=w766) -> ()  [unwired: 1 in, 2 out]
      }
      event "设置": Value Change {
        n508 = event-data() -> ()  [unwired: 1 in, 6 out]
        n509 = property on="窗格" class="Pane"("Origin"=T2 {"Horizontal"=0, "Vertical"=628} ("原点")) -> ()  [unwired: 2 in, 2 out]
      }
      event "pH", "DO", "Turb", "Cond", "Temp", "叶绿素a启用", "藻密度", "VISA资源名称", "连接方式", "IP", "Port", "自动断线重连", "水样测量时间": Value Change {
        n510 = event-data() -> ()  [unwired: 1 in, 6 out]
        n511 = flat-sequence {
          frame #0 {
            n512 = global write "断电保存变量.vi" "IP"("IP") -> ()
            n513 = global write "断电保存变量.vi" "Temp"("Temp") -> ()
            n514 = global write "断电保存变量.vi" "pH"("pH") -> ()
            n515 = global write "断电保存变量.vi" "藻密度"("藻密度") -> ()
            n516 = global write "断电保存变量.vi" "Cond"("Cond") -> ()
            n517 = global write "断电保存变量.vi" "连接方式"("连接方式") -> ()
            n518 = global write "断电保存变量.vi" "DO"("DO") -> ()
            n519 = global write "断电保存变量.vi" "Turb"("Turb") -> ()
            n520 = global write "断电保存变量.vi" "Port"("Port") -> ()
            n521 = global write "断电保存变量.vi" "叶绿素a启用"("叶绿素a启用") -> ()
            n522 = global write "断电保存变量.vi" "VISA资源名称"("VISA资源名称") -> ()
            n523 = global write "断电保存变量.vi" "水样测定时间"("水样测量时间") -> ()
            n524 = local read "自动断线重连"() -> (w769:bool)
            n525 = global write "断电保存变量.vi" "自动断线重连"(w769) -> ()
          }
          frame #1 {
            n526 = call <vilib>:"Application Directory.vi"() -> ("Application Directory"=w790:path)
            n527 = Build Path(base path=w790, name or relative path="data\\set.ini" ("名称或相对路径")) -> (appended path=w789:path)
            n528 = call <vilib>:"Open Config Data.vi"("configuration file path"=w789) -> ("error out"=w793:errorcluster, "refnum"=w794:T20)  [unwired: 8 in, 1 out]
            n529 = vi-ref "断电保存变量.vi"() -> (w787:refnum<vi>)
            n530 = call <userlib>:"Write Panel to INI__ogtk.vi"("error in (no error)"=w793, "VI ref"=w787, "refnum"=w794) -> ("error out"=w791:errorcluster, "refnum out"=w792:T20)  [unwired: 7 in]
            n531 = call <vilib>:"Close Config Data.vi"("error in (no error)"=w791, "refnum"=w792) -> ("error out"=w783:errorcluster, "file path"=w784:path)  [unwired: 8 in]
            n532 = Open/Create/Replace File(file path (use dialog)=w784, error in=w783) -> (refnum out=w785:refnum<file>, error out=w786:errorcluster)  [unwired: 4 in, 1 out]
            n533 = Flush File(refnum=w785, error in=w786) -> (refnum out=w781:refnum<file>, error out=w782:errorcluster)
            n534 = Close File(refnum=w781, error in=w782) -> ()  [unwired: 2 out]
          }
          frame #2 {
          }
        }
      }
      event "打开modbus": Value Change {
        n535 = event-data() -> ()  [unwired: 1 in, 6 out]
        n536 = global read "多参数全局变量.vi" "MB session in"() -> (w801:refnum<class "MB_Master.lvclass">)
        n537 = Flush Queue(queue=w796) -> (queue out=w795:refnum<queue>)  [unwired: 1 in, 2 out]
        n538 = property class="MB_Master"(reference=w801) -> ("Properties:Session Valid"=w800:bool)  [unwired: 1 in, 2 out]
        n539 = Select(t="close" ("元素"), s=w800, f="open" ("元素")) -> (s? t:f=w797:string)
        n540 = Enqueue Element(queue=w795, element=w797) -> ()  [unwired: 2 in, 3 out]
      }
      event "探头校正返回", "设置页返回": Value Change {
        n541 = event-data() -> ()  [unwired: 1 in, 6 out]
        n542 = property on="窗格" class="Pane"("Origin"=T2 {"Horizontal"=0, "Vertical"=0} ("原点")) -> ()  [unwired: 2 in, 2 out]
      }
      event "探头校正", "水温校准": Value Change {
        n543 = event-data() -> ()  [unwired: 1 in, 6 out]
        n544 = property on="窗格" class="Pane"("Origin"=T2 {"Horizontal"=1656, "Vertical"=0} ("原点")) -> ()  [unwired: 2 in, 2 out]
        n545 = vi-ref "水温校准.vi"() -> (w803:refnum<vi>)
        n546 = property class="VI"(reference=w803) -> (reference out=w805:refnum<vi>, "Exec.State"=w804:T7)  [unwired: 1 in, 1 out]
        n547 = case shown="\"Bad\", 默认" w804 {
          tunnel: [w809 w811] -> w807
          tunnel: w805 -> [w809 w810]
          frame "Bad", Default {
          }
          frame "Idle" {
            n548 = invoke class="VI" method="Run VI"(reference=w810, "Wait until done"=FALSE ("结束前等待"), "Auto Dispose Ref"=FALSE ("自动销毁引用")) -> (reference out=w811:refnum<vi>)  [unwired: 2 in, 4 out]
          }
        }
        n549 = invoke on="探头校准子面板" class="SubPnl" method="Remove VI"() -> (error out=w806:errorcluster)  [unwired: 3 in, 2 out]
        n550 = invoke on="探头校准子面板" class="SubPnl" method="Insert VI"(error in=w806, "VI Ref"=w807) -> ()  [unwired: 2 in, 4 out]
      }
      event "pH校准": Value Change {
        n551 = event-data() -> ()  [unwired: 1 in, 6 out]
        n552 = global read "断电保存变量.vi" "探头选择"() -> (w819:T5)
        n553 = Unbundle By Name(w819) -> ("pH探头选择"=w818:u16)
        n554 = case shown="2" w818 {
          tunnel: [w823 w824 w825] -> w817
          frame 0, Default {
            n555 = vi-ref "斯坦道多参数.lvlib:禹山pH校准.vi"() -> (w823:refnum<vi>)
          }
          frame 1 {
            n556 = vi-ref "斯坦道多参数.lvlib:pH电极校准.vi"() -> (w824:refnum<vi>)
          }
          frame 2 {
            n557 = vi-ref "斯坦道多参数.lvlib:纳清pH电极校准.vi"() -> (w825:refnum<vi>)
          }
        }
        n558 = property class="VI"(reference=w817) -> (reference out=w821:refnum<vi>, "Exec.State"=w820:T7)  [unwired: 1 in, 1 out]
        n559 = case shown="\"Bad\", 默认" w820 {
          tunnel: w821 -> [w826 w830]
          tunnel: [w826 w827] -> w815
          frame "Bad", Default {
          }
          frame "Idle" {
            n560 = invoke class="VI" method="Run VI"(reference=w830, "Wait until done"=FALSE ("结束前等待"), "Auto Dispose Ref"=FALSE ("自动销毁引用")) -> (reference out=w827:refnum<vi>)  [unwired: 2 in, 4 out]
          }
        }
        n561 = global read "多参数全局变量.vi" "校准VI引用句柄"() -> (w816:T21)
        n562 = invoke on="探头校准子面板" class="SubPnl" method="Remove VI"() -> (error out=w822:errorcluster)  [unwired: 3 in, 2 out]
        n563 = invoke on="探头校准子面板" class="SubPnl" method="Insert VI"(error in=w822, "VI Ref"=w815) -> ()  [unwired: 2 in, 4 out]
        n564 = Bundle By Name(cluster=w816, "pH校准VI引用句柄"=w815) -> (w814:T21)
        n565 = global write "多参数全局变量.vi" "校准VI引用句柄"(w814) -> ()
      }
      event "电导率校准": Value Change {
        n566 = event-data() -> ()  [unwired: 1 in, 6 out]
        n567 = global read "断电保存变量.vi" "探头选择"() -> (w836:T5)
        n568 = Unbundle By Name(w836) -> ("电导率探头选择"=w835:u16)
        n569 = case shown="2" w835 {
          tunnel: [w840 w841 w842] -> w834
          frame 0, Default {
            n570 = vi-ref "斯坦道多参数.lvlib:禹山电导率校准.vi"() -> (w840:refnum<vi>)
          }
          frame 1 {
            n571 = vi-ref "斯坦道多参数.lvlib:电导率电极校准.vi"() -> (w841:refnum<vi>)
          }
          frame 2 {
            n572 = vi-ref "斯坦道多参数.lvlib:纳清电导率电极校准.vi"() -> (w842:refnum<vi>)
          }
        }
        n573 = property class="VI"(reference=w834) -> (reference out=w838:refnum<vi>, "Exec.State"=w837:T7)  [unwired: 1 in, 1 out]
        n574 = case shown="\"Bad\", 默认" w837 {
          tunnel: [w843 w845] -> w831
          tunnel: w838 -> [w843 w844]
          frame "Bad", Default {
          }
          frame "Idle" {
            n575 = invoke class="VI" method="Run VI"(reference=w844, "Wait until done"=FALSE ("结束前等待"), "Auto Dispose Ref"=FALSE ("自动销毁引用")) -> (reference out=w845:refnum<vi>)  [unwired: 2 in, 4 out]
          }
        }
        n576 = global read "多参数全局变量.vi" "校准VI引用句柄"() -> (w833:T21)
        n577 = invoke on="探头校准子面板" class="SubPnl" method="Remove VI"() -> (error out=w839:errorcluster)  [unwired: 3 in, 2 out]
        n578 = Bundle By Name(cluster=w833, "COND校准VI引用句柄"=w831) -> (w832:T21)
        n579 = invoke on="探头校准子面板" class="SubPnl" method="Insert VI"(error in=w839, "VI Ref"=w831) -> ()  [unwired: 2 in, 4 out]
        n580 = global write "多参数全局变量.vi" "校准VI引用句柄"(w832) -> ()
      }
      event "溶解氧校准": Value Change {
        n581 = event-data() -> ()  [unwired: 1 in, 6 out]
        n582 = global read "断电保存变量.vi" "探头选择"() -> (w853:T5)
        n583 = Unbundle By Name(w853) -> ("DO探头选择"=w852:u16)
        n584 = case shown="2" w852 {
          tunnel: [w857 w858 w859] -> w851
          frame 0, Default {
            n585 = vi-ref "斯坦道多参数.lvlib:禹山溶解氧校准.vi"() -> (w857:refnum<vi>)
          }
          frame 1 {
            n586 = vi-ref "斯坦道多参数.lvlib:溶解氧电极校准.vi"() -> (w858:refnum<vi>)
          }
          frame 2 {
            n587 = vi-ref "斯坦道多参数.lvlib:纳清DO电极校准.vi"() -> (w859:refnum<vi>)
          }
        }
        n588 = property class="VI"(reference=w851) -> (reference out=w855:refnum<vi>, "Exec.State"=w854:T7)  [unwired: 1 in, 1 out]
        n589 = case shown="\"Bad\", 默认" w854 {
          tunnel: [w860 w862] -> w848
          tunnel: w855 -> [w860 w861]
          frame "Bad", Default {
          }
          frame "Idle" {
            n590 = invoke class="VI" method="Run VI"(reference=w861, "Wait until done"=FALSE ("结束前等待"), "Auto Dispose Ref"=FALSE ("自动销毁引用")) -> (reference out=w862:refnum<vi>)  [unwired: 2 in, 4 out]
          }
        }
        n591 = global read "多参数全局变量.vi" "校准VI引用句柄"() -> (w850:T21)
        n592 = invoke on="探头校准子面板" class="SubPnl" method="Remove VI"() -> (error out=w856:errorcluster)  [unwired: 3 in, 2 out]
        n593 = Bundle By Name(cluster=w850, "DO校准VI引用句柄"=w848) -> (w849:T21)
        n594 = invoke on="探头校准子面板" class="SubPnl" method="Insert VI"(error in=w856, "VI Ref"=w848) -> ()  [unwired: 2 in, 4 out]
        n595 = global write "多参数全局变量.vi" "校准VI引用句柄"(w849) -> ()
      }
      event "浊度校准": Value Change {
        n596 = event-data() -> ()  [unwired: 1 in, 6 out]
        n597 = global read "断电保存变量.vi" "探头选择"() -> (w870:T5)
        n598 = Unbundle By Name(w870) -> ("浊度探头选择"=w869:u16)
        n599 = case shown="2" w869 {
          tunnel: [w874 w875 w876] -> w868
          frame 0, Default {
            n600 = vi-ref "斯坦道多参数.lvlib:禹山浊度校准.vi"() -> (w874:refnum<vi>)
          }
          frame 1 {
            n601 = vi-ref "斯坦道多参数.lvlib:浊度电极校准.vi"() -> (w875:refnum<vi>)
          }
          frame 2 {
            n602 = vi-ref "斯坦道多参数.lvlib:纳清浊度电极校准.vi"() -> (w876:refnum<vi>)
          }
        }
        n603 = property class="VI"(reference=w868) -> (reference out=w872:refnum<vi>, "Exec.State"=w871:T7)  [unwired: 1 in, 1 out]
        n604 = case shown="\"Bad\", 默认" w871 {
          tunnel: [w877 w879] -> w865
          tunnel: w872 -> [w877 w878]
          frame "Bad", Default {
          }
          frame "Idle" {
            n605 = invoke class="VI" method="Run VI"(reference=w878, "Wait until done"=FALSE ("结束前等待"), "Auto Dispose Ref"=FALSE ("自动销毁引用")) -> (reference out=w879:refnum<vi>)  [unwired: 2 in, 4 out]
          }
        }
        n606 = global read "多参数全局变量.vi" "校准VI引用句柄"() -> (w867:T21)
        n607 = invoke on="探头校准子面板" class="SubPnl" method="Remove VI"() -> (error out=w873:errorcluster)  [unwired: 3 in, 2 out]
        n608 = invoke on="探头校准子面板" class="SubPnl" method="Insert VI"(error in=w873, "VI Ref"=w865) -> ()  [unwired: 2 in, 4 out]
        n609 = Bundle By Name(cluster=w867, "TURB校准VI引用句柄"=w865) -> (w866:T21)
        n610 = global write "多参数全局变量.vi" "校准VI引用句柄"(w866) -> ()
      }
      event "叶绿素a校准": Value Change {
        n611 = event-data() -> ()  [unwired: 1 in, 6 out]
        n612 = global read "断电保存变量.vi" "探头选择"() -> (w886:T5)
        n613 = Unbundle By Name(w886) -> ("叶绿素a探头选择"=w885:u16)
        n614 = case shown="2" w885 {
          tunnel: [w891 _ w892] -> w887
          frame 0, Default {
            n615 = vi-ref "禹山叶绿素a校准.vi"() -> (w891:refnum<vi>)
          }
          frame 1 {
          }
          frame 2 {
            n616 = vi-ref "斯坦道多参数.lvlib:纳清叶绿素a电极校准.vi"() -> (w892:refnum<vi>)
          }
        }
        n617 = property class="VI"(reference=w887) -> (reference out=w889:refnum<vi>, "Exec.State"=w888:T7)  [unwired: 1 in, 1 out]
        n618 = case shown="\"Bad\", 默认" w888 {
          tunnel: [w893 w895] -> w882
          tunnel: w889 -> [w893 w894]
          frame "Bad", Default {
          }
          frame "Idle" {
            n619 = invoke class="VI" method="Run VI"(reference=w894, "Wait until done"=FALSE ("结束前等待"), "Auto Dispose Ref"=FALSE ("自动销毁引用")) -> (reference out=w895:refnum<vi>)  [unwired: 2 in, 4 out]
          }
        }
        n620 = global read "多参数全局变量.vi" "校准VI引用句柄"() -> (w884:T21)
        n621 = invoke on="探头校准子面板" class="SubPnl" method="Remove VI"() -> (error out=w890:errorcluster)  [unwired: 3 in, 2 out]
        n622 = invoke on="探头校准子面板" class="SubPnl" method="Insert VI"(error in=w890, "VI Ref"=w882) -> ()  [unwired: 2 in, 4 out]
        n623 = Bundle By Name(cluster=w884, "CHLA校准VI引用句柄"=w882) -> (w883:T21)
        n624 = global write "多参数全局变量.vi" "校准VI引用句柄"(w883) -> ()
      }
      event "藻密度校准": Value Change {
        n625 = event-data() -> ()  [unwired: 1 in, 6 out]
        n626 = global read "断电保存变量.vi" "探头选择"() -> (w902:T5)
        n627 = Unbundle By Name(w902) -> ("蓝绿藻探头选择"=w901:u16)
        n628 = case shown="2" w901 {
          tunnel: [_ w907] -> w903
          frame 0, Default {
          }
          frame 2 {
            n629 = vi-ref "斯坦道多参数.lvlib:纳清蓝绿藻电极校准.vi"() -> (w907:refnum<vi>)
          }
        }
        n630 = property class="VI"(reference=w903) -> (reference out=w905:refnum<vi>, "Exec.State"=w904:T7)  [unwired: 1 in, 1 out]
        n631 = case shown="\"Bad\", 默认" w904 {
          tunnel: [w908 w910] -> w898
          tunnel: w905 -> [w908 w909]
          frame "Bad", Default {
          }
          frame "Idle" {
            n632 = invoke class="VI" method="Run VI"(reference=w909, "Wait until done"=FALSE ("结束前等待"), "Auto Dispose Ref"=FALSE ("自动销毁引用")) -> (reference out=w910:refnum<vi>)  [unwired: 2 in, 4 out]
          }
        }
        n633 = global read "多参数全局变量.vi" "校准VI引用句柄"() -> (w900:T21)
        n634 = invoke on="探头校准子面板" class="SubPnl" method="Remove VI"() -> (error out=w906:errorcluster)  [unwired: 3 in, 2 out]
        n635 = invoke on="探头校准子面板" class="SubPnl" method="Insert VI"(error in=w906, "VI Ref"=w898) -> ()  [unwired: 2 in, 4 out]
        n636 = Bundle By Name(cluster=w900, "BGA校准VI引用句柄"=w898) -> (w899:T21)
        n637 = global write "多参数全局变量.vi" "校准VI引用句柄"(w899) -> ()
      }
    }
  }
  n638 = while {
    tunnel: w11 -> [w914]
    tunnel: w1 -> [_]
    stop <- FALSE stop-if-true
    n639 = Dequeue Element(queue=w914) -> (element=w913:string)  [unwired: 2 in, 3 out]
    n640 = case shown="\"open\"" w913 {
      tunnel: [_ w916 w926] -> _
      frame "假", Default {
      }
      frame "open" {
        n641 = global read "多参数全局变量.vi" "MB session in"() -> (w921:refnum<class "MB_Master.lvclass">)
        n642 = global read "断电保存变量.vi" "VISA资源名称"() -> (w923:refnum<visa-resource-name>)
        n643 = global read "断电保存变量.vi" "连接方式"() -> (w919:u16)
        n644 = call "close MB.vi"("MB session in"=w921) -> ("error out"=w924:errorcluster)  [unwired: 10 in]
        n645 = global read "断电保存变量.vi" "Port"() -> (w917:u16)
        n646 = global read "断电保存变量.vi" "IP"() -> (w918:string)
        n647 = call "open MB.vi"("Port (502)"=w917, "IP Address"=w918, "MODE"=w919, "error in (no error)"=w924, "Serial Config"=T23 {"baud rate (bps)"=9600, "stop bits"=10, "parity"=0, "flow control"=0, "timeout"=1000, "retries"=1}, "VISA资源名称"=w923) -> ("error out"=w916:errorcluster, "MB session out"=w920:refnum<class "MB_Master.lvclass">)  [unwired: 4 in]
        n648 = global write "多参数全局变量.vi" "MB session in"(w920) -> ()
      }
      frame "close" {
        n649 = global read "多参数全局变量.vi" "MB session in"() -> (w925:refnum<class "MB_Master.lvclass">)
        n650 = call "close MB.vi"("MB session in"=w925) -> ("error out"=w926:errorcluster)  [unwired: 10 in]
      }
    }
  }
  n651 = while {
    tunnel: w11 -> [w928]
    stop <- FALSE stop-if-true
    # "断线重连"
    n652 = global read "断电保存变量.vi" "连接方式"() -> (w929:u16)
    n653 = Wait (ms)(milliseconds to wait=u32 10000 ("等待时间（毫秒）")) -> ()  [unwired: 1 out]
    n654 = case shown="1" w929 {
      tunnel: w928 -> [_ w932]
      frame 0, Default {
      }
      frame 1 {
        n655 = case shown="真" "自动断线重连" {
          tunnel: w932 -> [_ w935]
          frame False {
          }
          frame True {
            n656 = global read "多参数全局变量.vi" "MB session in"() -> (w934:refnum<class "MB_Master.lvclass">)
            n657 = property class="MB_Master"(reference=w934) -> ("Properties:Session Valid"=w933:bool)  [unwired: 1 in, 2 out]
            n658 = case shown="假" w933 {
              tunnel: w935 -> [w936 _]
              frame False {
                n659 = Flush Queue(queue=w936) -> (queue out=w938:refnum<queue>)  [unwired: 1 in, 2 out]
                n660 = Enqueue Element(queue=w938, element="open" ("元素")) -> ()  [unwired: 2 in, 3 out]
              }
              frame True {
              }
            }
          }
        }
      }
    }
  }
